vi "Station Detail Main.vi"(8 "error in (no error)":errorcluster, 11 "LineScan in":refnum<class "LineScan.lvclass">) -> (0 "error out":errorcluster, 2 "Station Out":T1=enum."ImformOut", 3 "LineScan out":refnum<class "LineScan.lvclass">)   [LabVIEW 2019, in "LineScan.lvclass"]
uses:
  LineScan.lvclass
  Ctrl/Station Action.ctl
  Ctrl/ProjectStepSelect.ctl
  Ctrl/StationCmdSelect.ctl
  Ctrl/Auto Inspection Station Name2.ctl
  Ctrl/Auto Inspection Data Name.ctl
  Ctrl/S2 Station IO.ctl
  Ctrl/MeasureDisplayTab.ctl
  Ctrl/Table Save.ctl
  Ctrl/ModbusCmd.ctl
  Ctrl/S2 Station Input.ctl
  Global/Process Global.vi
  LLB/Commonly VI/Main Glb.vi
  Ctrl/ProjectCmdStep.ctl
  BarcodeScan/Ctl/Board Scan IO.ctl
  Laser Detect/Ctl/S11 Station IO.ctl
  LLB/Commonly VI.lvlib
panel:
  out "data":dbl
  out "data 2":bool
  out "Array":string[](array[string])
  out "Blue Scan receive":string
  out "S1 ChkSum":string
  out "S1 ToolStringOut":string
  out "ToolStringOut_P1_2":string
  out "ToolStringOut_P1":string
  out "Initial_ChkSum":string
  out "ToolStringOut_Init":string
  out "CurrentCmd 2":string
  out "retry次數 2":string[](array[string])
  out "Retry 2":i32
  out "Program1 receive 2":string
  out "Initial receive 2":string
  out "T2 buffer":string
  out "T2 μA":dbl format="%#_6f"
  out "T1 μA":dbl format="%#_6f"
  out "T1 buffer":string
  out "S2 receive":string
  out "Blue Scan2 receive":string
  out "S1 receive":string
  out "Initial receive":string
  out "CurrentCmd":string
  out "Act Step":i32
  out "present":i32
  out "format receive":string
  out "Retry":i32
  out "subarray":string[](array[string])
  out "retry次數":string[](array[string])
  in  "Table Control":string[][](table)=[["PCBA BARCODE", ""], ["硬體(Tool初始化)", ""], ["company(Tool初始化)", ""], ["耗電流 uA(電流表)", "T"], ["電池負載電壓", "T"], ["晶片ID(Tool FORMAT)", "F"], ["雷雕ID(TOOl scan、藍芽接收器)", "S"], ["Format(Tool FORMAT)", "F"], ["Programe(Tool Programe)", "P"]]
  out "Numeric":dbl
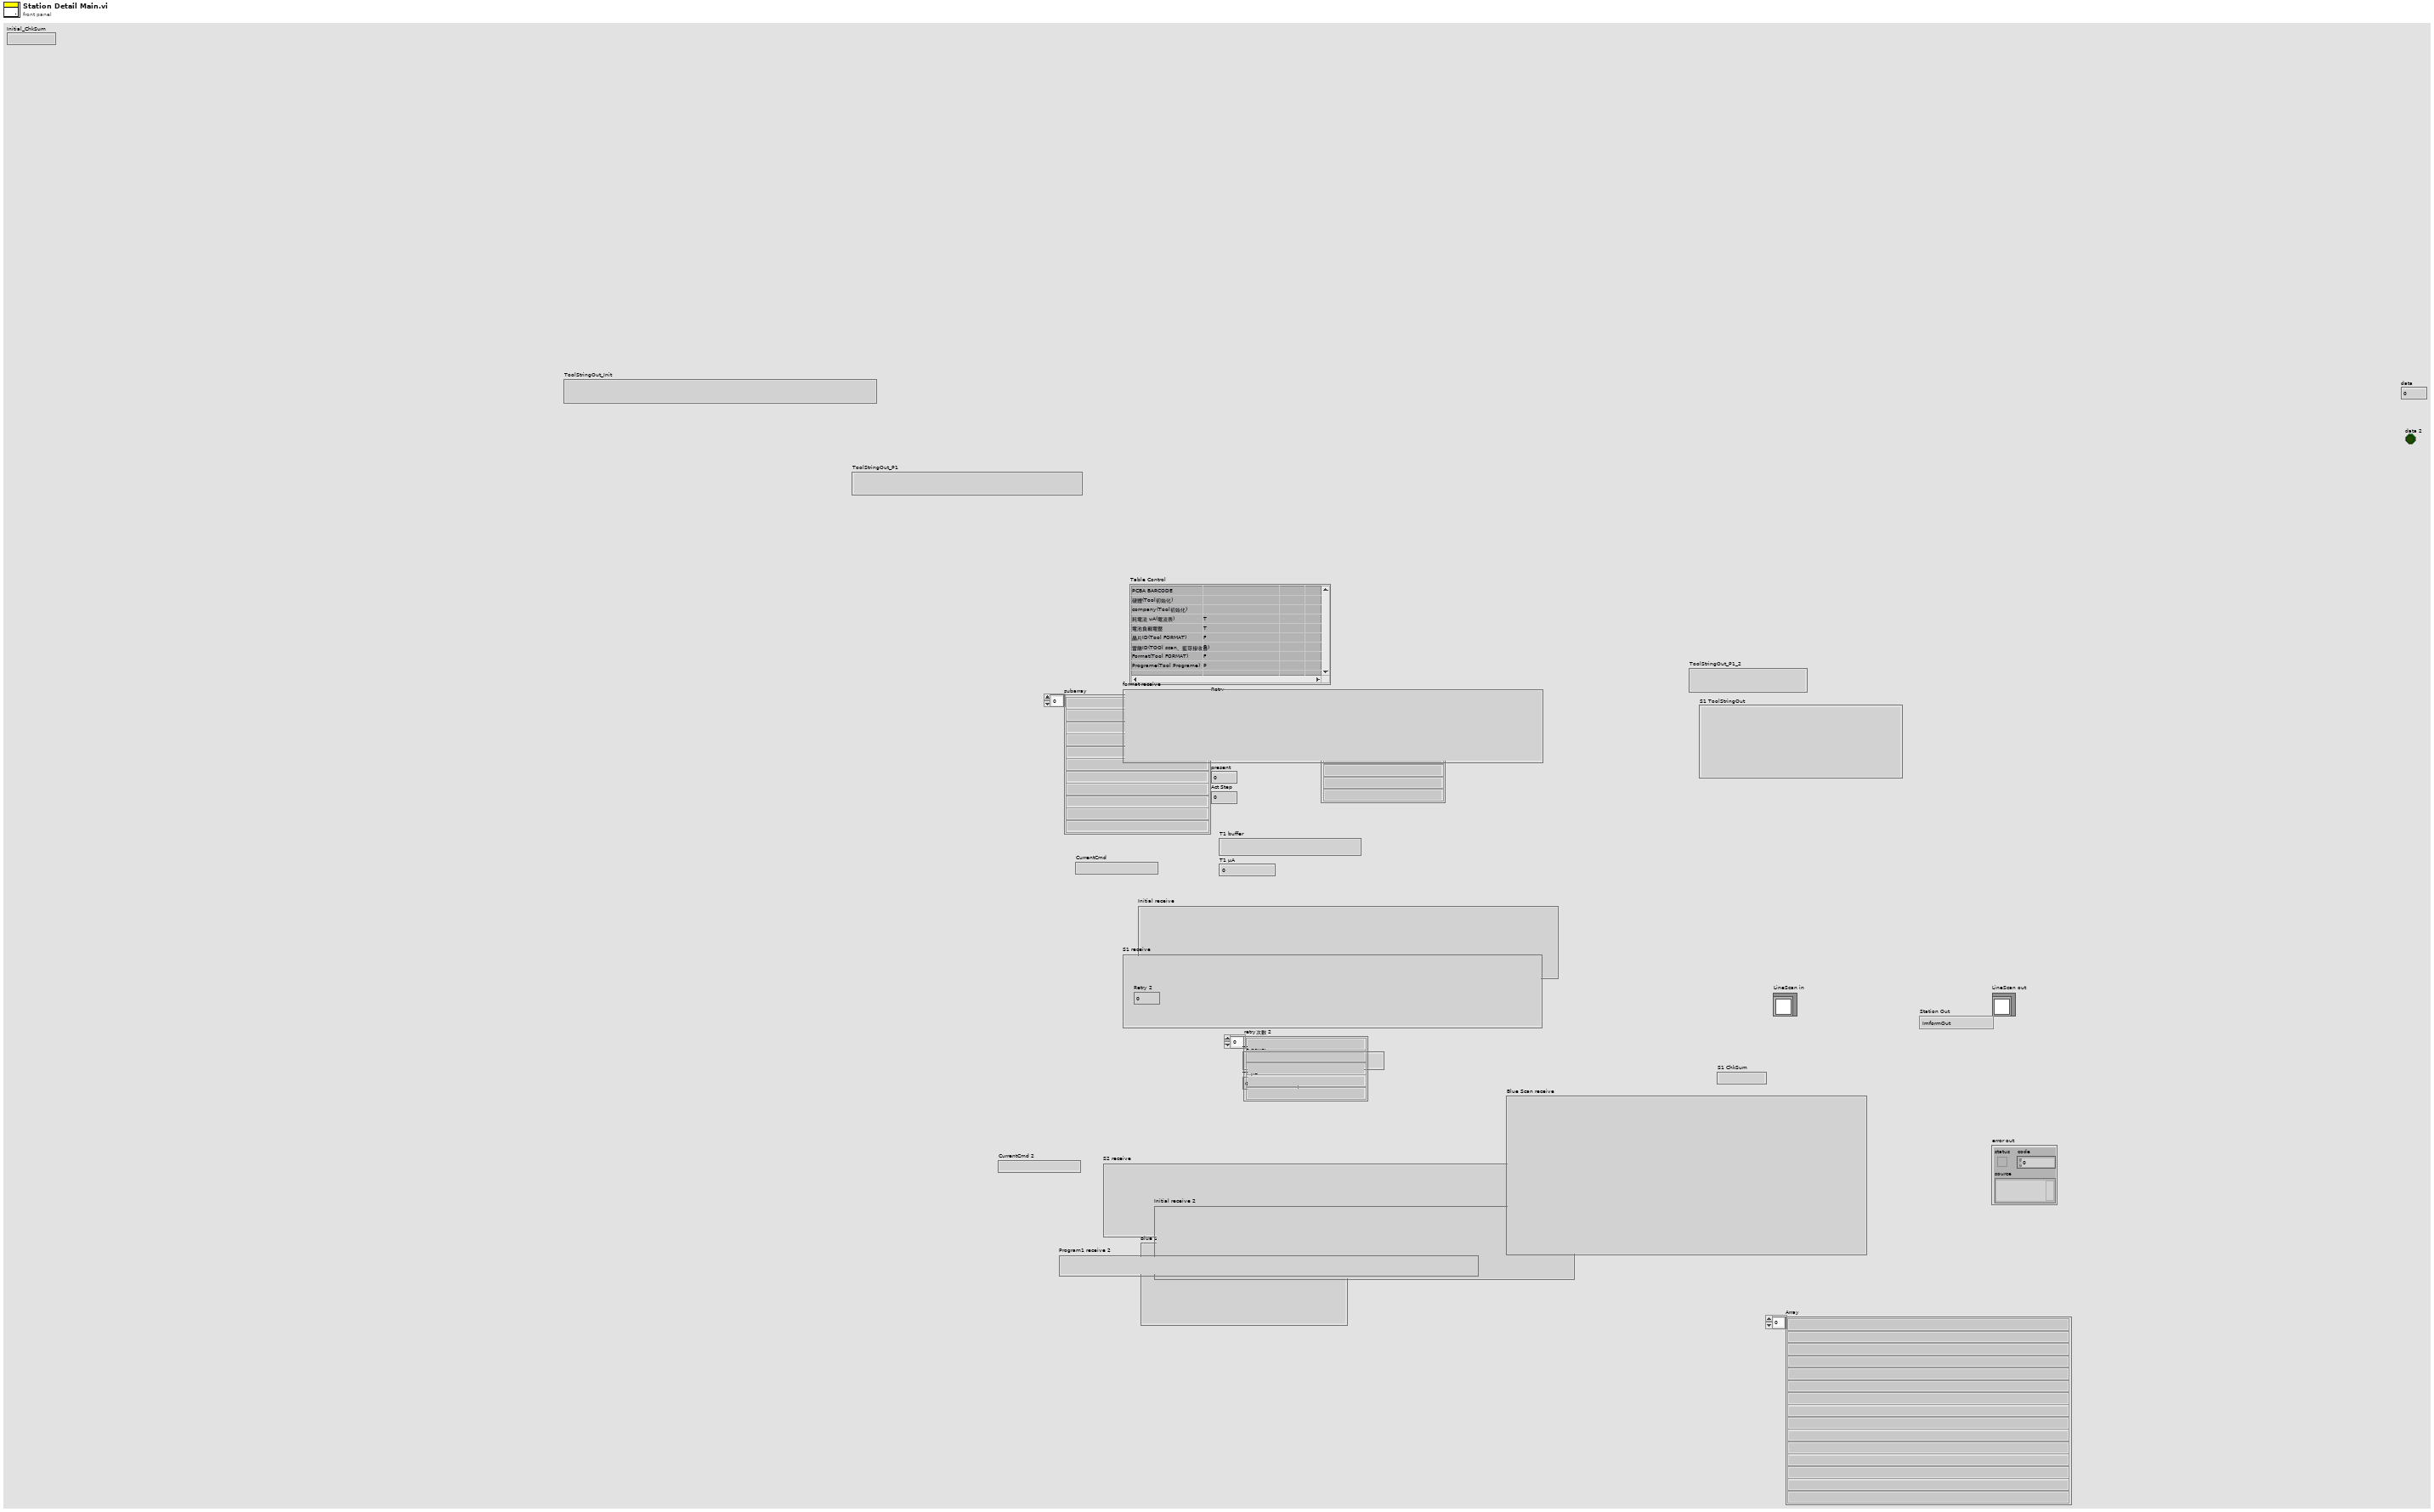
[diagram p1: front panel]
types:
  T1 = typedef "Station Action.ctl" = enum16{"Wait Item In", "Dectect Action", "ImformOut"}
  T2 = cluster{"starting address":u16, "number of inputs":u16, "Sat Coils":bool[], "Holding Registers":u16[]}
  T3 = typedef "ModbusCmd.ctl" = enum16{"Connect", "Disconnect", "Init", "Fetch Basic Objects", "Fetch Input Refisters", "Fetch Discrete Inputs", "Set Coils", "Set Holding Registers", "Write Single Holding", "Exit"}
  T4 = typedef "Board Scan IO.ctl" = enum16{"S1 Barcode Scan", "S1 載盤條碼比對OK", "S1 載盤條碼比對NG", "S1PLC 條碼可讀取訊號", "S1備用_04", "S1備用_05", "S1備用_06", "S1備用_07", "S1備用_08", "S1 發送條碼完成"}
  T5 = typedef "S2 Station IO.ctl" = enum16{"S2站PC動作中_20", "電流量測完成產品OK_21", "電流量測完成產品NG_22", "S2站Format 執行_23", "S2 Format OK_24", "S2 Format NG_25", "S2站燒入執行_26", "S2站燒入OK_27", "S2站燒入NG_28", "S2站動作完成_29", "S3 PC動作中_30", "S3 Format 此站執行_31", "S3 Format OK_32", "S3 Format NG_33", "S3 燒入程式 此站執行_34", "S3 燒入程式 OK_35", "S3 燒入程式 NG_36", "S3 備用_37", "S3 備用_38", "S3 動作完成_39", "S4 PC動作中_40", "S4 量測完成 產品正常_41", "S4 量測完成 產品NG_42", "S4 Format 此站執行_43", "S4 Format OK_44", "S4 Format NG_45", "S4 燒入 此站不執行_46", "S4 燒入程式 OK_47", "S4 燒入程式 NG_48", "S4 藍芽Scan OK_49", "S4 藍芽Scan NG_50", "S4 動作完成_51", "給PLC要量電流訊號", "給PLC要量電壓訊號"}
  T6 = typedef "S11 Station IO.ctl" = enum16{"S11雷射測量動作中", "S11雷射測點1完成", "S11雷射測點2完成", "S11雷測測量OK", "S11雷測測量NG", "S11雷測測量重測", "S11備用_6", "S11備用_7", "S11備用_8", "S11雷射測高完成"}
  T7 = typedef "StationCmdSelect.ctl" = enum16{"Action", "Command", "Return", "DTime", "Retry"}
  T8 = typedef "Auto Inspection Data Name.ctl" = enum16{"LocalRun", "ItemSN(TimeCode)", "CurrentAction", "Error", "Data", "OKNG", "電壓值", "電壓值判斷", "電流值", "電流值判斷", "Laser1 Data", "Laser2 Data", "Laser OKNG", "StationNO"}
  T9 = typedef "Auto Inspection Station Name2.ctl" = enum16{"S1Barcode", "S2Measure", "S3Measure", "S4Measure", "S5Measure", "S11_LaserCheck", "S8_Vision AI"}
  T10 = typedef "Table Save.ctl" = enum16{"initial", "Add", "Write", "Replace", "Delete", "REad", "RedTable", "Load"}
  T11 = typedef "MeasureDisplayTab.ctl" = enum16{"Tray Barcode", "PCBA BARCODE", "硬體(Tool初始化)", "company(Tool初始化)", "耗電流 uA(電流表)", "電池負載電壓", "晶片ID(Tool FORMAT)", "雷雕ID(TOOl scan、藍芽接收器)", "Format(Tool FORMAT)", "Programe(Tool Programe)", "MAC(藍芽接收器)", "ID(藍芽接收器)", "KPA(藍芽接收器)", "溫度(藍芽接收器)", "SENSOR電池電壓(藍芽接收器)", "RSSI(藍芽接收器)", "SensorType_315(FSK scan)", "FSKsnVol_315(FSK scan)", "FSKscanl_315(FSK scan)", "P_315(FSK scan)", "T_315(FSK scan)", "SensorType_433(ASK scan)", "ASKsnVol_433(ASK scan)", "ASKscan_433(ASK scan)", "P_433(ASK scan)", "T_433(ASK scan)", "測高Data"}
  T12 = typedef "S2 Station Input.ctl" = enum16{"00PLC Alive clock", "01PLC狀態(手動)", "02PLC狀態(自動)", "03PLC Alarm", "04備用", "05備用", "06備用", "07備用", "08備用", "09備用", "10載盤有料for條碼", "11_備用", "12_備用", "13_備用", "14_備用", "15_備用", "16_備用", "17_備用", "18_備用", "19_備用", "20_載盤有料訊號ForS2站", "21_PLC下達可測電流訊號", "22_PLC下達可測電壓訊號"}
  T13 = typedef "ProjectStepSelect.ctl" = enum16{"ProjectName", "Name", "Initial", "Reset", "Format", "Program1", "Program2", "Scan", "Finish", "MToolWork", "DataCheck", "DataSave", "OutputPLC", "WaitInputS1", "WaitInputOff"}
  T14 = typedef "ProjectCmdStep.ctl" = enum16{"Project Name", "commamd1", "commamd2", "commamd3", "wat time1", "return1", "return2", "return3", "wat time2", "over time", "retry"}
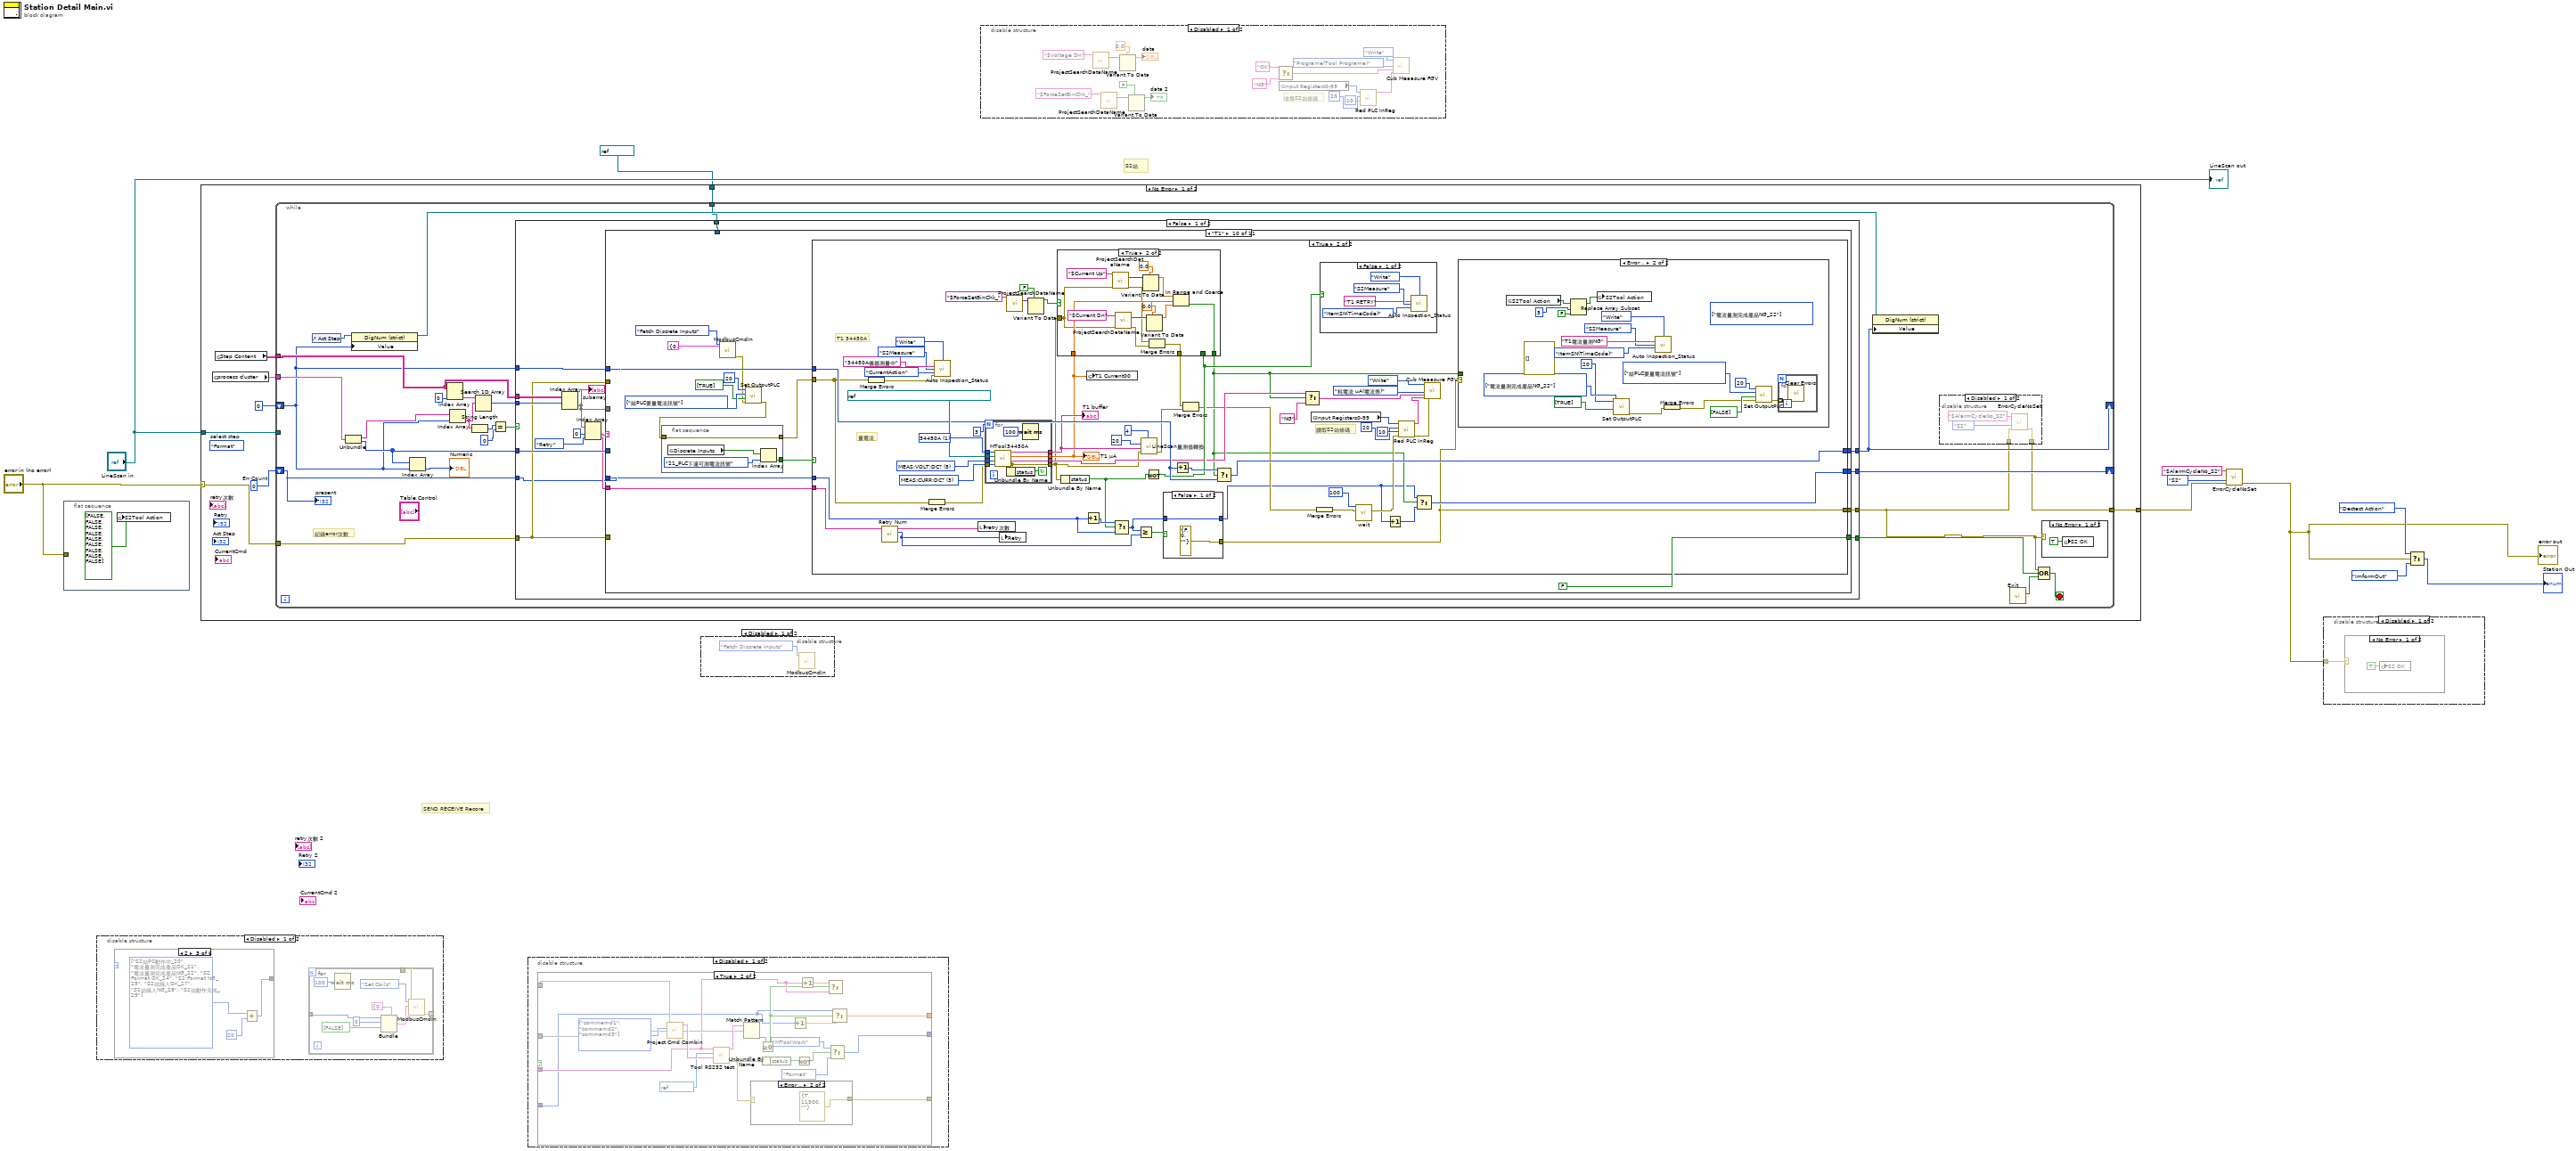
[diagram p0: block diagram]
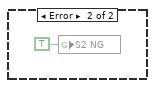
[diagram p2: hidden frame]
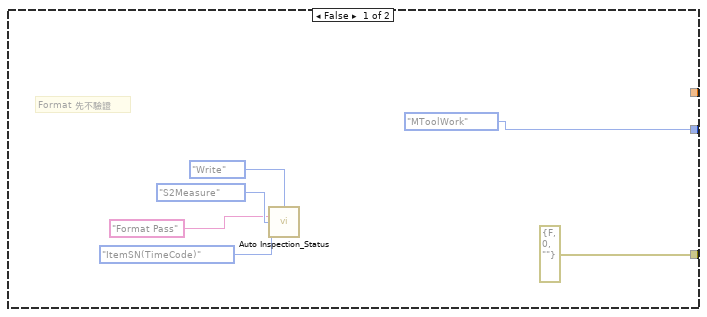
[diagram p6: hidden frame]
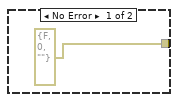
[diagram p7: hidden frame]
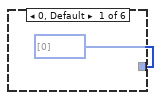
[diagram p9: hidden frame]
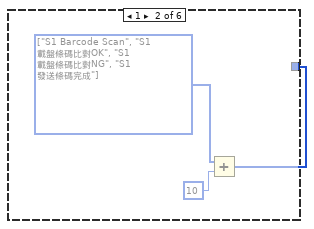
[diagram p10: hidden frame]
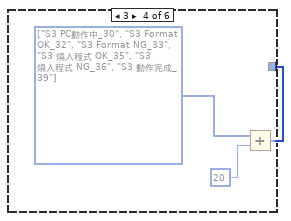
[diagram p11: hidden frame]
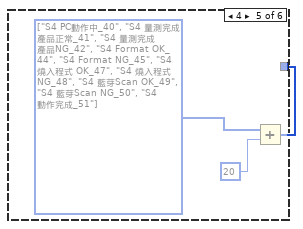
[diagram p12: hidden frame]
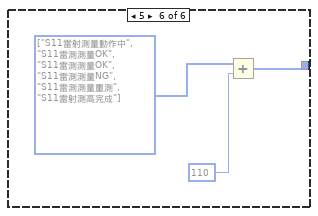
[diagram p13: hidden frame]
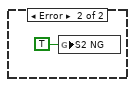
[diagram p15: hidden frame]
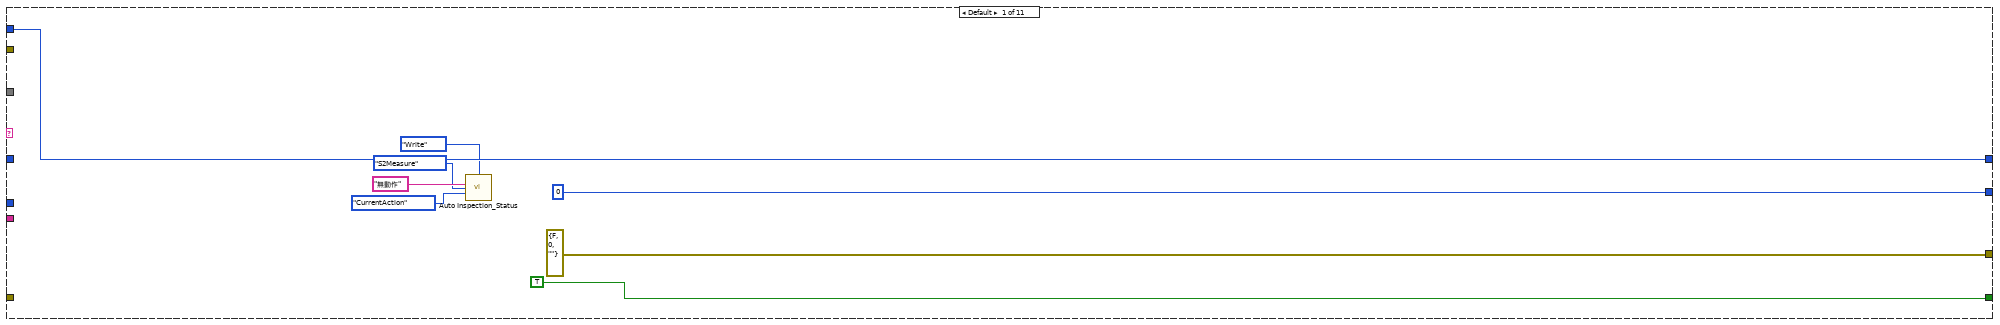
[diagram p17: hidden frame]
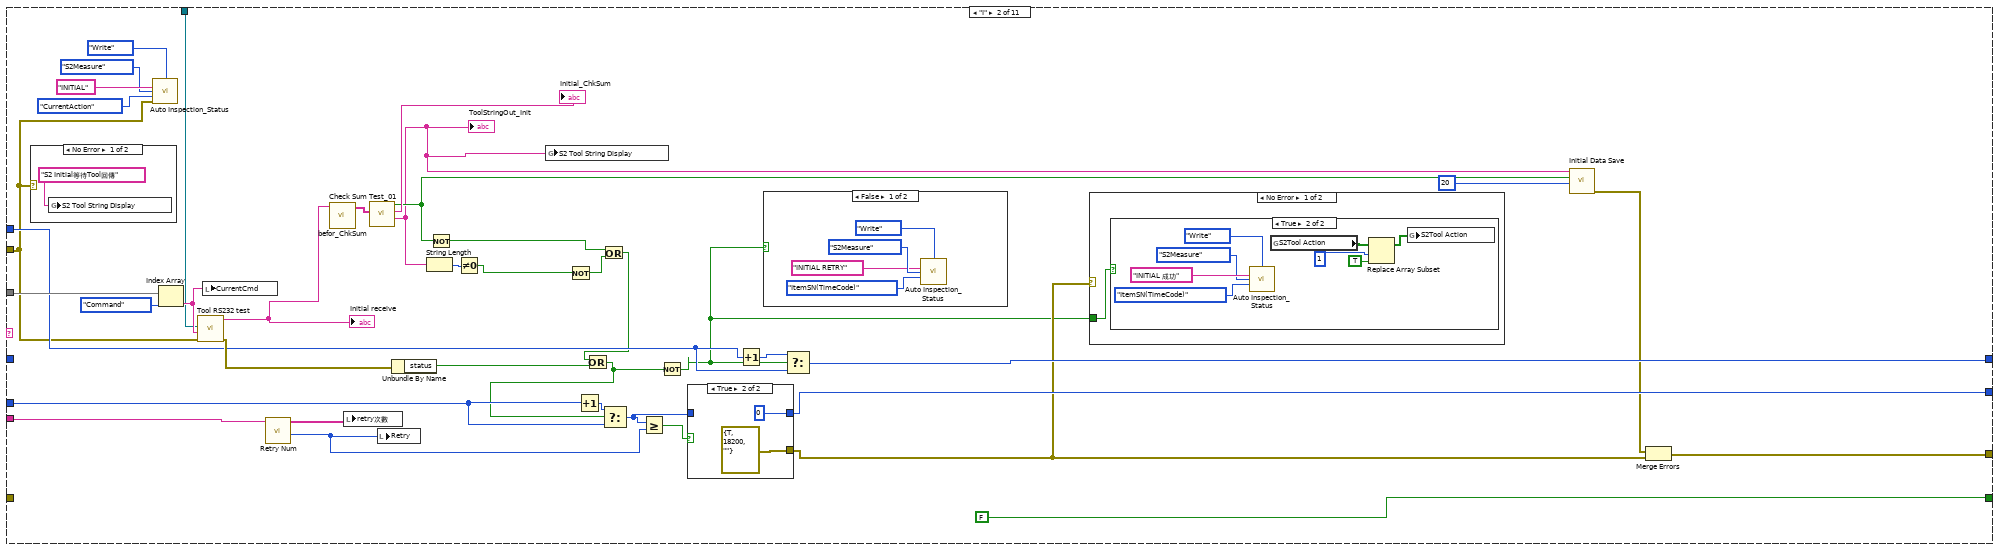
[diagram p18: hidden frame]
diagram:
  # "S2站"
  # "SEND RECEIVE Recore"
  n1 = flat-sequence {
    tunnel: "error in (no error)" -> [_]
    frame #0 {
      n2 = global write "Process Global.vi" "S2Tool Action"(bool[] [FALSE, FALSE, FALSE, FALSE, FALSE, FALSE, FALSE, FALSE, FALSE] ("S2Tool Action")) -> ()
    }
  }
  n3 = disable-structure shown="Disabled" {
    frame Disabled {
      n4 = case shown="2" {
        selector: _ -> [_ _ _ _ _ _]
        tunnel: [i32[] [0] w22 w25 w28 w31 w34] -> _
        frame 0, Default {
        }
        frame 1 {
          w24 = T4[] [enum."S1 Barcode Scan", enum."S1 載盤條碼比對OK", enum."S1 載盤條碼比對NG", enum."S1 發送條碼完成"] items=["S1 Barcode Scan", "S1 載盤條碼比對OK", "S1 載盤條碼比對NG", "S1PLC 條碼可讀取訊號", "S1備用_04", "S1備用_05", "S1備用_06", "S1備用_07", "S1備用_08", "S1 發送條碼完成"]
          n5 = Add(x=w24, y=10) -> (x+y=w22:i32[])
        }
        frame 2 {
          w26 = T5[] [enum."S2站PC動作中_20", enum."電流量測完成產品OK_21", enum."電流量測完成產品NG_22", enum."S2 Format OK_24", enum."S2 Format NG_25", enum."S2站燒入OK_27", enum."S2站燒入NG_28", enum."S2站動作完成_29"] items=["S2站PC動作中_20", "電流量測完成產品OK_21", "電流量測完成產品NG_22", "S2站Format 執行_23", "S2 Format OK_24", "S2 Format NG_25", "S2站燒入執行_26", "S2站燒入OK_27", "S2站燒入NG_28", "S2站動作完成_29", "S3 PC動作中_30", "S3 Format 此站執行_31", "S3 Format OK_32", "S3 Format NG_33", "S3 燒入程式 此站執行_34", "S3 燒入程式 OK_35", "S3 燒入程式 NG_36", "S3 備用_37", "S3 備用_38", "S3 動作完成_39", "S4 PC動作中_40", "S4 量測完成 產品正常_41", "S4 量測完成 產品NG_42", "S4 Format 此站執行_43", "S4 Format OK_44", "S4 Format NG_45", "S4 燒入 此站不執行_46", "S4 燒入程式 OK_47", "S4 燒入程式 NG_48", "S4 藍芽Scan OK_49", "S4 藍芽Scan NG_50", "S4 動作完成_51", "給PLC要量電流訊號", "給PLC要量電壓訊號"]
          n6 = Add(x=w26, y=20) -> (x+y=w25:i32[])
        }
        frame 3 {
          w29 = T5[] [enum."S3 PC動作中_30", enum."S3 Format OK_32", enum."S3 Format NG_33", enum."S3 燒入程式 OK_35", enum."S3 燒入程式 NG_36", enum."S3 動作完成_39"] items=["S2站PC動作中_20", "電流量測完成產品OK_21", "電流量測完成產品NG_22", "S2站Format 執行_23", "S2 Format OK_24", "S2 Format NG_25", "S2站燒入執行_26", "S2站燒入OK_27", "S2站燒入NG_28", "S2站動作完成_29", "S3 PC動作中_30", "S3 Format 此站執行_31", "S3 Format OK_32", "S3 Format NG_33", "S3 燒入程式 此站執行_34", "S3 燒入程式 OK_35", "S3 燒入程式 NG_36", "S3 備用_37", "S3 備用_38", "S3 動作完成_39", "S4 PC動作中_40", "S4 量測完成 產品正常_41", "S4 量測完成 產品NG_42", "S4 Format 此站執行_43", "S4 Format OK_44", "S4 Format NG_45", "S4 燒入 此站不執行_46", "S4 燒入程式 OK_47", "S4 燒入程式 NG_48", "S4 藍芽Scan OK_49", "S4 藍芽Scan NG_50", "S4 動作完成_51", "給PLC要量電流訊號", "給PLC要量電壓訊號"]
          n7 = Add(x=w29, y=20) -> (x+y=w28:i32[])
        }
        frame 4 {
          w32 = T5[] [enum."S4 PC動作中_40", enum."S4 量測完成 產品正常_41", enum."S4 量測完成 產品NG_42", enum."S4 Format OK_44", enum."S4 Format NG_45", enum."S4 燒入程式 OK_47", enum."S4 燒入程式 NG_48", enum."S4 藍芽Scan OK_49", enum."S4 藍芽Scan NG_50", enum."S4 動作完成_51"] items=["S2站PC動作中_20", "電流量測完成產品OK_21", "電流量測完成產品NG_22", "S2站Format 執行_23", "S2 Format OK_24", "S2 Format NG_25", "S2站燒入執行_26", "S2站燒入OK_27", "S2站燒入NG_28", "S2站動作完成_29", "S3 PC動作中_30", "S3 Format 此站執行_31", "S3 Format OK_32", "S3 Format NG_33", "S3 燒入程式 此站執行_34", "S3 燒入程式 OK_35", "S3 燒入程式 NG_36", "S3 備用_37", "S3 備用_38", "S3 動作完成_39", "S4 PC動作中_40", "S4 量測完成 產品正常_41", "S4 量測完成 產品NG_42", "S4 Format 此站執行_43", "S4 Format OK_44", "S4 Format NG_45", "S4 燒入 此站不執行_46", "S4 燒入程式 OK_47", "S4 燒入程式 NG_48", "S4 藍芽Scan OK_49", "S4 藍芽Scan NG_50", "S4 動作完成_51", "給PLC要量電流訊號", "給PLC要量電壓訊號"]
          n8 = Add(x=w32, y=20) -> (x+y=w31:i32[])
        }
        frame 5 {
          w35 = T6[] [enum."S11雷射測量動作中", enum."S11雷測測量OK", enum."S11雷測測量OK", enum."S11雷測測量NG", enum."S11雷測測量重測", enum."S11雷射測高完成"] items=["S11雷射測量動作中", "S11雷射測點1完成", "S11雷射測點2完成", "S11雷測測量OK", "S11雷測測量NG", "S11雷測測量重測", "S11備用_6", "S11備用_7", "S11備用_8", "S11雷射測高完成"]
          n9 = Add(x=w35, y=110) -> (x+y=w34:i32[])
        }
      }
      n10 = for {
        tunnel: [w14] -> _ mode=indexing
        tunnel: _ -> [w13]
        tunnel: _ -> [w12] mode=indexing
        n11 = Wait (ms)(milliseconds to wait=100) -> ()  [unwired: 1 out]
        n12 = Bundle(cluster=T2 {"starting address"=0, "number of inputs"=0, "Sat Coils"=[], "Holding Registers"=[]} ("data"), "starting address"=w12, "number of inputs"=u16 0, "Sat Coils"=bool[] [FALSE]) -> (w17:T2)  [unwired: 1 in]
        n13 = call "ModbusCmdIn.vi"("error in (no error)"=w13, "data"=w17, "Enum"=ModbusCmd."Set Coils") -> ("error out"=w14:errorcluster)  [unwired: 8 in]
      }
    }
    frame Enabled {
    }
  }
  n14 = case shown="No Error" "error in (no error)" {
    selector: "error in (no error)" -> [w38 w854]
    tunnel: [w44 w854] -> w2
    tunnel: "LineScan in" -> [w43 _]
    tunnel: refnum<visa-resource-name> "COM1" ("VISA resource name") -> [w37 _]
    frame No Error {
      w39 = 0  # Err Count
      (unwired) ProjectStepSelect."Format"  # select step
      n15 = global read "Process Global.vi" "process cluster"() -> (w41:cluster{string[], i32[]})
      n16 = global read "Process Global.vi" "Step Content"() -> (w42:string[][])
      n17 = while {
        tunnel: [w45] -> w44
        shift-right: [w52] -> _
        shift-left: 0 -> [w53]
        tunnel: w43 -> [_]
        shift-right: [w49] -> _
        shift-left: w39 -> [w55]
        tunnel: w42 -> [w66]
        tunnel: w41 -> [w65]
        tunnel: w38 -> [w50]
        tunnel: w37 -> [w48]
        stop <- w67 stop-if-true
        # "紀錄error次數"
        n18 = control-ref of="Act Step"() -> (w54:refnum<vi>)
        n19 = Unbundle(w65) -> (w68:string[], w69:i32[])
        n20 = property class="DigNum (strict)"(reference=w54, "Value"=w53) -> (reference out=w51:refnum<vi>)  [unwired: 1 in, 1 out]
        n21 = Index Array(array=w69, index=w53) -> (element=→"Numeric":i32)
        n22 = Index Array(array=w66, index (col)=0 ("disabled index (col)")) -> (element=w63:string[])  [unwired: 1 in]
        n23 = Index Array(array=w68, index=w53) -> (element=w59:string)
        n24 = String Length(string=w59) -> (length=w60:i32)
        n25 = Search 1D Array(1D array=w63, element=w59) -> (index of element=w62:i32)  [unwired: 1 in]
        n26 = Equal?(x=w60, y=0) -> (x = y?=w57:bool)
        n27 = case shown="False" w57 {
          tunnel: w69 -> [w92 _]
          tunnel: w66 -> [w91 _]
          tunnel: w62 -> [w90 _]
          tunnel: [w81 TRUE] -> w56
          tunnel: [w83 errorcluster {"status"=FALSE, "code"=0, "source"=""} ("error constant")] -> w46
          tunnel: w53 -> [w85 _]
          tunnel: [w84 w851] -> w52
          tunnel: w55 -> [w79 _]
          tunnel: w50 -> [w80 _]
          tunnel: [w78 w851] -> w49
          tunnel: w48 -> [w77 _]
          frame False {
            n28 = Index Array(array=w91, index (row)=w90) -> (element=w86:string[])  [unwired: 1 in]
            "subarray" <- w86
            n29 = Index Array(array=w86, index #1=0 ("index"), index #2=StationCmdSelect."Retry") -> (element #1=w88:string, element #2=w87:string)
            n30 = case shown="\"T1\"" w88 {
              tunnel: w92 -> [_ _ _ _ _ _ _ _ w583 _ _]
              tunnel: w87 -> [_ w129 w176 w244 w340 w394 w493 w537 _ w599 w753]
              tunnel: w86 -> [_ w130 w177 w243 w342 w397 w492 w538 _ _ _]
              tunnel: w85 -> [w100 w113 w178 w239 w341 w396 w468 w540 w578 w598 w755]
              tunnel: [w100 w128 w175 w241 w339 w393 w494 w536 w577 w597 w754] -> w84
              tunnel: [errorcluster {"status"=FALSE, "code"=0, "source"=""} ("error constant") w106 w168 w227 w300 w390 w485 w533 errorcluster {"status"=FALSE, "code"=0, "source"=""} ("error constant") w596 w752] -> w83
              tunnel: [TRUE FALSE FALSE FALSE FALSE FALSE FALSE FALSE FALSE FALSE FALSE] -> w81
              tunnel: w80 -> [_ _ _ _ _ _ _ _ _ _ _]
              tunnel: w80 -> [_ w102 w167 w218 w298 w389 w456 w539 _ _ _]
              tunnel: w79 -> [_ w121 w171 w221 w324 w395 w470 w517 _ w594 w751]
              tunnel: [0 ("Err Count") w122 w172 w222 w325 w392 w471 w518 0 ("Err Count") w595 w750] -> w78
              tunnel: w77 -> [_ w120 w169 w220 w314 w398 w469 w516 _ _ _]
              frame Default {
                n31 = call "Auto Inspection_Status.vi"("Action"=enum16{"Initial", "Write", "Read"}."Write", "DataIn"="無動作", "Station"=Auto_Inspection_Station_Name2."S2Measure", "Data"=Auto_Inspection_Data_Name."CurrentAction") -> ()  [unwired: 9 in, 3 out]
              }
              frame "I" {
                n32 = case shown="No Error" w102 {
                  frame No Error {
                    n33 = global write "Process Global.vi" "S2 Tool String Display"("S2 Initial等待Tool回傳" ("S2 Tool String Display")) -> ()
                  }
                  frame Error {
                  }
                }
                n34 = call "Auto Inspection_Status.vi"("Action"=enum16{"Initial", "Write", "Read"}."Write", "DataIn"="INITIAL", "Station"=Auto_Inspection_Station_Name2."S2Measure", "Data"=Auto_Inspection_Data_Name."CurrentAction", "error in"=w102) -> ()  [unwired: 8 in, 3 out]
                n35 = Index Array(array=w130, index=StationCmdSelect."Command") -> (element=w132:string)
                n36 = call "Tool RS232 test.vi"("error in (no error)"=w102, "Cmd In"=w132, "VISA resource name"=w120) -> ("error out"=w139:errorcluster, "receive string"=w105:string)  [unwired: 7 in]
                "Initial receive" <- w105
                n37 = local write "CurrentCmd"(w132) -> ()
                n38 = call "Retry Num.vi"("String"=w129) -> ("Numeric"=w136:i32, "retry次數"=w133:string[])  [unwired: 9 in]
                n39 = call "befor_ChkSum.vi"("ToolString Input"=w105) -> ("Array"=w115:string[])  [unwired: 9 in, 1 out]
                n40 = local write "retry次數"(w133) -> ()
                n41 = call "Check Sum Test_01.vi"("Array"=w115) -> ("ToolStringOut_01"=w104:string, "ChkSum"=→"Initial_ChkSum":string, "x = y?"=w109:bool)  [unwired: 8 in]
                "ToolStringOut_Init" <- w104
                n42 = local write "Retry"(w136) -> ()
                n43 = Unbundle By Name(w139) -> ("status"=w112:bool)
                n44 = String Length(string=w104) -> (length=w118:i32)
                n45 = Not(x=w109) -> (.not. x?=w116:bool)
                n46 = Not Equal To 0?(x=w118) -> (x != 0?=w119:bool)
                n47 = global write "Process Global.vi" "S2 Tool String Display"(w104) -> ()
                n48 = Not(x=w119) -> (.not. x?=w117:bool)
                n49 = Increment(x=w121) -> (x+1=w137:i32)
                n50 = Or(x=w116, y=w117) -> (x .or. y?=w111:bool)
                n51 = Or(x=w111, y=w112) -> (x .or. y?=w110:bool)
                n52 = Select(t=w137, s=w110, f=w121) -> (s? t:f=w134:i32)
                n53 = Greater Or Equal?(x=w134, y=w136) -> (x >= y?=w135:bool)
                n54 = Not(x=w110) -> (.not. x?=w101:bool)
                n55 = case shown="True" w135 {
                  tunnel: [errorcluster {"status"=FALSE, "code"=0, "source"=""} ("error constant") errorcluster {"status"=TRUE, "code"=18200, "source"=""} ("error constant")] -> w103
                  tunnel: w134 -> [w162 _]
                  tunnel: [w162 0] -> w122
                  frame False {
                  }
                  frame True {
                  }
                }
                n56 = Increment(x=w113) -> (x+1=w138:i32)
                n57 = case shown="False" w101 {
                  frame False {
                    n58 = call "Auto Inspection_Status.vi"("Action"=enum16{"Initial", "Write", "Read"}."Write", "DataIn"="INITIAL RETRY", "Station"=Auto_Inspection_Station_Name2."S2Measure", "Data"=Auto_Inspection_Data_Name."ItemSN(TimeCode)") -> ()  [unwired: 9 in, 3 out]
                  }
                  frame True {
                  }
                }
                n59 = Select(t=w138, s=w101, f=w113) -> (s? t:f=w128:i32)
                n60 = case shown="No Error" w103 {
                  tunnel: w101 -> [w145 _]
                  frame No Error {
                    n61 = case shown="True" w145 {
                      frame False {
                      }
                      frame True {
                        n62 = call "Auto Inspection_Status.vi"("Action"=enum16{"Initial", "Write", "Read"}."Write", "DataIn"="INITIAL 成功", "Station"=Auto_Inspection_Station_Name2."S2Measure", "Data"=Auto_Inspection_Data_Name."ItemSN(TimeCode)") -> ()  [unwired: 9 in, 3 out]
                        n63 = global read "Process Global.vi" "S2Tool Action"() -> (w149:bool[])
                        n64 = Replace Array Subset(array=w149, new element=TRUE ("new element/subarray"), index=1) -> (w146:bool[])
                        n65 = global write "Process Global.vi" "S2Tool Action"(w146) -> ()
                      }
                    }
                  }
                  frame Error {
                    n66 = call "Auto Inspection_Status.vi"("Action"=enum16{"Initial", "Write", "Read"}."Write", "DataIn"="INITIAL 失敗 ", "Station"=Auto_Inspection_Station_Name2."S2Measure", "Data"=Auto_Inspection_Data_Name."ItemSN(TimeCode)") -> ()  [unwired: 9 in, 3 out]
                    n67 = global read "Process Global.vi" "S2Tool Action"() -> (w157:bool[])
                    n68 = Replace Array Subset(array=w157, new element=FALSE ("new element/subarray"), index=1) -> (w154:bool[])
                    n69 = global write "Process Global.vi" "S2Tool Action"(w154) -> ()
                  }
                }
                n70 = call "Initial Data Save.vi"("index"=20, "OK and NG"=w109, "String In"=w104) -> ("error out"=w107:errorcluster)  [unwired: 8 in]
                n71 = Merge Errors(w107, w103) -> (w106:errorcluster)
              }
              frame "R" {
                n72 = call "Auto Inspection_Status.vi"("Action"=enum16{"Initial", "Write", "Read"}."Write", "DataIn"="RESET", "Station"=Auto_Inspection_Station_Name2."S2Measure", "Data"=Auto_Inspection_Data_Name."CurrentAction", "error in"=w167) -> ()  [unwired: 8 in, 3 out]
                n73 = call "Retry Num.vi"("String"=w176) -> ("Numeric"=w186:i32, "retry次數"=w185:string[])  [unwired: 9 in]
                n74 = Index Array(array=w177, index=StationCmdSelect."Command") -> (element=w184:string)
                n75 = local write "retry次數"(w185) -> ()
                n76 = call "Tool RS232 test.vi"("error in (no error)"=w167, "Cmd In"=w184, "VISA resource name"=w169) -> ("error out"=w190:errorcluster, "receive string"=→"Initial receive 2":string)  [unwired: 7 in]
                n77 = local write "CurrentCmd"(w184) -> ()
                n78 = local write "Retry"(w186) -> ()
                n79 = Unbundle By Name(w190) -> ("status"=w188:bool)
                n80 = Increment(x=w171) -> (x+1=w187:i32)
                n81 = Not(x=w188) -> (.not. x?=w166:bool)
                n82 = Select(t=w187, s=w188, f=w171) -> (s? t:f=w173:i32)
                n83 = Greater Or Equal?(x=w173, y=w186) -> (x >= y?=w170:bool)
                n84 = case shown="True" w170 {
                  tunnel: [errorcluster {"status"=FALSE, "code"=0, "source"=""} ("error constant") errorcluster {"status"=TRUE, "code"=18207, "source"=""} ("error constant")] -> w168
                  tunnel: w173 -> [w213 w215]
                  tunnel: [w213 w215] -> w172
                  frame False {
                  }
                  frame True {
                  }
                }
                n85 = case shown="False" w166 {
                  frame False {
                    n86 = call "Auto Inspection_Status.vi"("Action"=enum16{"Initial", "Write", "Read"}."Write", "DataIn"="RESET RETRY ", "Station"=Auto_Inspection_Station_Name2."S2Measure", "Data"=Auto_Inspection_Data_Name."ItemSN(TimeCode)") -> ()  [unwired: 9 in, 3 out]
                  }
                  frame True {
                  }
                }
                n87 = Increment(x=w178) -> (x+1=w189:i32)
                n88 = Select(t=w189, s=w166, f=w178) -> (s? t:f=w175:i32)
                n89 = case shown="No Error" w168 {
                  tunnel: w166 -> [w196 _]
                  frame No Error {
                    n90 = case shown="True" w196 {
                      frame False {
                      }
                      frame True {
                        n91 = call "Auto Inspection_Status.vi"("Action"=enum16{"Initial", "Write", "Read"}."Write", "DataIn"="RESET 成功 ", "Station"=Auto_Inspection_Station_Name2."S2Measure", "Data"=Auto_Inspection_Data_Name."ItemSN(TimeCode)") -> ()  [unwired: 9 in, 3 out]
                        n92 = global read "Process Global.vi" "S2Tool Action"() -> (w200:bool[])
                        n93 = Replace Array Subset(array=w200, new element=TRUE ("new element/subarray"), index=0) -> (w197:bool[])
                        n94 = global write "Process Global.vi" "S2Tool Action"(w197) -> ()
                      }
                    }
                  }
                  frame Error {
                    n95 = call "Auto Inspection_Status.vi"("Action"=enum16{"Initial", "Write", "Read"}."Write", "DataIn"="RESET 失敗 ", "Station"=Auto_Inspection_Station_Name2."S2Measure", "Data"=Auto_Inspection_Data_Name."ItemSN(TimeCode)") -> ()  [unwired: 9 in, 3 out]
                    n96 = global read "Process Global.vi" "S2Tool Action"() -> (w208:bool[])
                    n97 = Replace Array Subset(array=w208, new element=FALSE ("new element/subarray"), index=0) -> (w205:bool[])
                    n98 = global write "Process Global.vi" "S2Tool Action"(w205) -> ()
                  }
                }
              }
              frame "F" {
                # "SEND RECEIVE Recore"
                n99 = call "Retry Num.vi"("String"=w244) -> ("Numeric"=w235:i32, "retry次數"=w231:string[])  [unwired: 9 in]
                n100 = local write "retry次數"(w231) -> ()
                n101 = Index Array(array=w243, index=StationCmdSelect."Command") -> (element=w230:string)
                n102 = local write "Retry"(w235) -> ()
                n103 = call "Tool RS232 test.vi"("error in (no error)"=w218, "Cmd In"=w230, "VISA resource name"=w220) -> ("error out"=w240:errorcluster, "receive string"=→"format receive":string)  [unwired: 7 in]
                n104 = local write "CurrentCmd"(w230) -> ()
                n105 = Unbundle By Name(w240) -> ("status"=w237:bool)
                n106 = Not(x=w237) -> (.not. x?=w217:bool)
                n107 = call "Auto Inspection_Status.vi"("Action"=enum16{"Initial", "Write", "Read"}."Write", "DataIn"="FORMAT", "Station"=Auto_Inspection_Station_Name2."S2Measure", "Data"=Auto_Inspection_Data_Name."CurrentAction", "error in"=w218) -> ()  [unwired: 8 in, 3 out]
                n108 = Increment(x=w221) -> (x+1=w236:i32)
                n109 = Select(t=w236, s=w237, f=w221) -> (s? t:f=w232:i32)
                n110 = Increment(x=w239) -> (x+1=w238:i32)
                n111 = Greater Or Equal?(x=w232, y=w235) -> (x >= y?=w234:bool)
                n112 = Select(t=w238, s=w217, f=w239) -> (s? t:f=w241:i32)
                n113 = case shown="True" w234 {
                  tunnel: [errorcluster {"status"=FALSE, "code"=0, "source"=""} ("error constant") errorcluster {"status"=TRUE, "code"=18201, "source"=""} ("error constant")] -> w219
                  tunnel: w232 -> [w289 _]
                  tunnel: [w289 0] -> w222
                  frame False {
                  }
                  frame True {
                  }
                }
                n114 = case shown="False" w217 {
                  frame False {
                    n115 = call "Auto Inspection_Status.vi"("Action"=enum16{"Initial", "Write", "Read"}."Write", "DataIn"="FORMAT RETRY ", "Station"=Auto_Inspection_Station_Name2."S2Measure", "Data"=Auto_Inspection_Data_Name."ItemSN(TimeCode)") -> ()  [unwired: 9 in, 3 out]
                  }
                  frame True {
                  }
                }
                n116 = case shown="No Error" w219 {
                  tunnel: [w250 w286] -> w228
                  tunnel: w217 -> [w249 _]
                  frame No Error {
                    n117 = case shown="True" w249 {
                      tunnel: [_ w267] -> w250
                      frame False {
                      }
                      frame True {
                        w268 = T5[] [enum."S2站Format 執行_23", enum."S2 Format OK_24"] items=["S2站PC動作中_20", "電流量測完成產品OK_21", "電流量測完成產品NG_22", "S2站Format 執行_23", "S2 Format OK_24", "S2 Format NG_25", "S2站燒入執行_26", "S2站燒入OK_27", "S2站燒入NG_28", "S2站動作完成_29", "S3 PC動作中_30", "S3 Format 此站執行_31", "S3 Format OK_32", "S3 Format NG_33", "S3 燒入程式 此站執行_34", "S3 燒入程式 OK_35", "S3 燒入程式 NG_36", "S3 備用_37", "S3 備用_38", "S3 動作完成_39", "S4 PC動作中_40", "S4 量測完成 產品正常_41", "S4 量測完成 產品NG_42", "S4 Format 此站執行_43", "S4 Format OK_44", "S4 Format NG_45", "S4 燒入 此站不執行_46", "S4 燒入程式 OK_47", "S4 燒入程式 NG_48", "S4 藍芽Scan OK_49", "S4 藍芽Scan NG_50", "S4 動作完成_51", "給PLC要量電流訊號", "給PLC要量電壓訊號"]
                        # "收尋S2站條碼"
                        n118 = global read "Main Glb.vi" "Input Registers0-99"() -> (w255:u16[])
                        n119 = call "Set OutputPLC.vi"("Address In"=20, "Array 2"=w268, "Sat Coils"=bool[] [TRUE]) -> ("Error Out"=w267:errorcluster[])  [unwired: 7 in]
                        n120 = global read "Process Global.vi" "S2Tool Action"() -> (w262:bool[])
                        n121 = call "Red PLC InReg.vi"("length"=10, "index"=20, "Input Registers Arr"=w255) -> ("Rad In Reg"=w258:string)  [unwired: 7 in, 1 out]
                        n122 = call "Cub Meaasure FGV.vi"("Action"=Table_Save."Write" ("Enum"), "Save Index"=MeasureDisplayTab."Format(Tool FORMAT)", "DataIn"="OK", "SN"=w258) -> ()  [unwired: 8 in, 8 out]
                        n123 = Replace Array Subset(array=w262, new element=TRUE ("new element/subarray"), index=2) -> (w259:bool[])
                        n124 = global write "Process Global.vi" "S2Tool Action"(w259) -> ()
                        n125 = call "Auto Inspection_Status.vi"("Action"=enum16{"Initial", "Write", "Read"}."Write", "DataIn"="FORMAT完成", "Station"=Auto_Inspection_Station_Name2."S2Measure", "Data"=Auto_Inspection_Data_Name."ItemSN(TimeCode)") -> ()  [unwired: 9 in, 3 out]
                      }
                    }
                  }
                  frame Error {
                    w288 = T5[] [enum."S2站Format 執行_23", enum."S2 Format NG_25"] items=["S2站PC動作中_20", "電流量測完成產品OK_21", "電流量測完成產品NG_22", "S2站Format 執行_23", "S2 Format OK_24", "S2 Format NG_25", "S2站燒入執行_26", "S2站燒入OK_27", "S2站燒入NG_28", "S2站動作完成_29", "S3 PC動作中_30", "S3 Format 此站執行_31", "S3 Format OK_32", "S3 Format NG_33", "S3 燒入程式 此站執行_34", "S3 燒入程式 OK_35", "S3 燒入程式 NG_36", "S3 備用_37", "S3 備用_38", "S3 動作完成_39", "S4 PC動作中_40", "S4 量測完成 產品正常_41", "S4 量測完成 產品NG_42", "S4 Format 此站執行_43", "S4 Format OK_44", "S4 Format NG_45", "S4 燒入 此站不執行_46", "S4 燒入程式 OK_47", "S4 燒入程式 NG_48", "S4 藍芽Scan OK_49", "S4 藍芽Scan NG_50", "S4 動作完成_51", "給PLC要量電流訊號", "給PLC要量電壓訊號"]
                    # "收尋S2站條碼"
                    n126 = global read "Main Glb.vi" "Input Registers0-99"() -> (w274:u16[])
                    n127 = call "Set OutputPLC.vi"("Address In"=20, "Array 2"=w288, "Sat Coils"=bool[] [TRUE]) -> ("Error Out"=w286:errorcluster[])  [unwired: 7 in]
                    n128 = call "Red PLC InReg.vi"("length"=10, "index"=20, "Input Registers Arr"=w274) -> ("Rad In Reg"=w277:string)  [unwired: 7 in, 1 out]
                    n129 = global read "Process Global.vi" "S2Tool Action"() -> (w281:bool[])
                    n130 = call "Cub Meaasure FGV.vi"("Action"=Table_Save."Write" ("Enum"), "Save Index"=MeasureDisplayTab."Format(Tool FORMAT)", "DataIn"="NG", "SN"=w277) -> ()  [unwired: 8 in, 8 out]
                    n131 = call "Auto Inspection_Status.vi"("Action"=enum16{"Initial", "Write", "Read"}."Write", "DataIn"="FORMAT 失敗 ", "Station"=Auto_Inspection_Station_Name2."S2Measure", "Data"=Auto_Inspection_Data_Name."ItemSN(TimeCode)") -> ()  [unwired: 9 in, 3 out]
                    n132 = Replace Array Subset(array=w281, new element=FALSE ("new element/subarray"), index=2) -> (w278:bool[])
                    n133 = global write "Process Global.vi" "S2Tool Action"(w278) -> ()
                  }
                }
                n134 = Merge Errors(w228, w219) -> (w227:errorcluster)
              }
              frame "P1" {
                # "經過燒錄後第二次Tool回傳"
                # "下Cmd後第一次Tool回傳"
                # "收尋S2站條碼"
                n135 = case shown="No Error" w298 {
                  frame No Error {
                    n136 = global write "Process Global.vi" "S2 Tool String Display"("S2燒錄 等待Tool回傳" ("S2 Tool String Display")) -> ()
                  }
                  frame Error {
                  }
                }
                n137 = call "Retry Num.vi"("String"=w340) -> ("Numeric"=w348:i32, "retry次數"=w345:string[])  [unwired: 9 in]
                n138 = Index Array(array=w342, index=StationCmdSelect."Command") -> (element=w344:string)
                n139 = local write "retry次數"(w345) -> ()
                n140 = call "Tool RS232 test.vi"("error in (no error)"=w298, "Cmd In"=w344, "VISA resource name"=w314) -> ("error out"=w315:errorcluster, "receive string"=w316:string)  [unwired: 7 in]
                n141 = local write "CurrentCmd"(w344) -> ()
                n142 = local write "Retry"(w348) -> ()
                n143 = call "befor_ChkSum.vi"("ToolString Input"=w316) -> ("Array"=w317:string[])  [unwired: 9 in, 1 out]
                n144 = call "Check Sum Test_01.vi"("Array"=w317) -> ("ToolStringOut_01"=w320:string, "x = y?"=w318:bool)  [unwired: 8 in, 1 out]
                "ToolStringOut_P1" <- w320
                n145 = call "Auto Inspection_Status.vi"("Action"=enum16{"Initial", "Write", "Read"}."Write", "DataIn"="PROGRAM1", "Station"=Auto_Inspection_Station_Name2."S2Measure", "Data"=Auto_Inspection_Data_Name."CurrentAction", "error in"=w298) -> ()  [unwired: 8 in, 3 out]
                n146 = String Length(string=w320) -> (length=w322:i32)
                n147 = Not(x=w318) -> (.not. x?=w319:bool)
                n148 = Not Equal To 0?(x=w322) -> (x != 0?=w323:bool)
                n149 = Not(x=w323) -> (.not. x?=w321:bool)
                n150 = Or(x=w319, y=w321) -> ()  [unwired: 1 out]
                n151 = call "ToolProgramTest.vi"("error in (no error)"=w315, "VISA resource name"=w314) -> ("Array"=w305:string[])  [unwired: 4 in, 5 out]
                n152 = Index Array(array=w305, index=0) -> (element=w312:string)
                n153 = call "befor_ChkSum.vi"("ToolString Input"=w312) -> ("Array"=w311:string[])  [unwired: 9 in, 1 out]
                n154 = call "Check Sum Test_01.vi"("Array"=w311) -> ("ToolStringOut_01"=w299:string, "x = y?"=w308:bool)  [unwired: 8 in, 1 out]
                "ToolStringOut_P1_2" <- w299
                n155 = global write "Process Global.vi" "S2 Tool String Display"(w299) -> ()
                n156 = String Length(string=w299) -> (length=w309:i32)
                n157 = Not(x=w308) -> (.not. x?=w307:bool)
                n158 = Unbundle By Name(w315) -> ("status"=w303:bool)
                n159 = call "Get ProgReturn Info.vi"("String"=w299) -> ("Chk OK or Fail"=w304:bool)  [unwired: 8 in, 2 out]
                n160 = Not Equal To 0?(x=w309) -> (x != 0?=w310:bool)
                n161 = Not(x=w310) -> (.not. x?=w306:bool)
                n162 = Compound Arithmetic op=OR(invert w304, w307, w306) -> (w302:bool)
                n163 = Or(x=w302, y=w303) -> (x .or. y?=w301:bool)
                n164 = Not(x=w301) -> (.not. x?=w297:bool)
                n165 = Increment(x=w324) -> (x+1=w349:i32)
                n166 = Select(t=w349, s=w301, f=w324) -> (s? t:f=w346:i32)
                n167 = case shown="False" w297 {
                  frame False {
                    n168 = call "Auto Inspection_Status.vi"("Action"=enum16{"Initial", "Write", "Read"}."Write", "DataIn"="PROGRAM1 RETRY", "Station"=Auto_Inspection_Station_Name2."S2Measure", "Data"=Auto_Inspection_Data_Name."ItemSN(TimeCode)") -> ()  [unwired: 9 in, 3 out]
                  }
                  frame True {
                  }
                }
                n169 = Select(t="OK" ("DataIn"), s=w304, f="NG" ("DataIn")) -> (s? t:f=w333:string)
                n170 = Greater Or Equal?(x=w346, y=w348) -> (x >= y?=w347:bool)
                n171 = global read "Main Glb.vi" "Input Registers0-99"() -> (w327:u16[])
                n172 = case shown="False" w347 {
                  tunnel: [errorcluster {"status"=FALSE, "code"=0, "source"=""} ("error constant") errorcluster {"status"=TRUE, "code"=18202, "source"=""} ("error constant")] -> w300
                  tunnel: w346 -> [w379 _]
                  tunnel: [w379 0] -> w325
                  frame False {
                  }
                  frame True {
                  }
                }
                n173 = call "Red PLC InReg.vi"("length"=10, "index"=20, "Input Registers Arr"=w327) -> ("Rad In Reg"=w294:string)  [unwired: 7 in, 1 out]
                n174 = Increment(x=w341) -> (x+1=w350:i32)
                n175 = call "Cub Meaasure FGV.vi"("Action"=Table_Save."Write" ("Enum"), "Save Index"=MeasureDisplayTab."Programe(Tool Programe)", "DataIn"=w333, "SN"=w294) -> ()  [unwired: 8 in, 8 out]
                n176 = Select(t=w350, s=w297, f=w341) -> (s? t:f=w339:i32)
                n177 = global write "Main Glb.vi" "S2 Barcode ID"(w294) -> ()
                n178 = call "Cub Meaasure FGV.vi"("Action"=Table_Save."REad" ("Enum"), "Save Index"=MeasureDisplayTab."Tray Barcode", "SN"=w294) -> ("Read Index Data"=w293:string)  [unwired: 9 in, 7 out]
                n179 = global write "Main Glb.vi" "S2 Tary ID"(w293) -> ()
                n180 = case shown="No Error" w300 {
                  tunnel: w297 -> [w356 _]
                  frame No Error {
                    n181 = case shown="True" w356 {
                      frame False {
                      }
                      frame True {
                        w366 = T5[] [enum."S2站燒入執行_26", enum."S2站燒入OK_27"] items=["S2站PC動作中_20", "電流量測完成產品OK_21", "電流量測完成產品NG_22", "S2站Format 執行_23", "S2 Format OK_24", "S2 Format NG_25", "S2站燒入執行_26", "S2站燒入OK_27", "S2站燒入NG_28", "S2站動作完成_29", "S3 PC動作中_30", "S3 Format 此站執行_31", "S3 Format OK_32", "S3 Format NG_33", "S3 燒入程式 此站執行_34", "S3 燒入程式 OK_35", "S3 燒入程式 NG_36", "S3 備用_37", "S3 備用_38", "S3 動作完成_39", "S4 PC動作中_40", "S4 量測完成 產品正常_41", "S4 量測完成 產品NG_42", "S4 Format 此站執行_43", "S4 Format OK_44", "S4 Format NG_45", "S4 燒入 此站不執行_46", "S4 燒入程式 OK_47", "S4 燒入程式 NG_48", "S4 藍芽Scan OK_49", "S4 藍芽Scan NG_50", "S4 動作完成_51", "給PLC要量電流訊號", "給PLC要量電壓訊號"]
                        n182 = global read "Process Global.vi" "S2Tool Action"() -> (w361:bool[])
                        n183 = call "Set OutputPLC.vi"("Address In"=20, "Array 2"=w366, "Sat Coils"=bool[] [TRUE]) -> ()  [unwired: 7 in, 1 out]
                        n184 = Replace Array Subset(array=w361, new element=TRUE ("new element/subarray"), index=3) -> (w358:bool[])
                        n185 = global write "Process Global.vi" "S2Tool Action"(w358) -> ()
                        n186 = call "Auto Inspection_Status.vi"("Action"=enum16{"Initial", "Write", "Read"}."Write", "DataIn"="PROGRAM1成功", "Station"=Auto_Inspection_Station_Name2."S2Measure", "Data"=Auto_Inspection_Data_Name."ItemSN(TimeCode)") -> ()  [unwired: 9 in, 3 out]
                      }
                    }
                  }
                  frame Error {
                    w378 = T5[] [enum."S2站燒入執行_26", enum."S2站燒入NG_28"] items=["S2站PC動作中_20", "電流量測完成產品OK_21", "電流量測完成產品NG_22", "S2站Format 執行_23", "S2 Format OK_24", "S2 Format NG_25", "S2站燒入執行_26", "S2站燒入OK_27", "S2站燒入NG_28", "S2站動作完成_29", "S3 PC動作中_30", "S3 Format 此站執行_31", "S3 Format OK_32", "S3 Format NG_33", "S3 燒入程式 此站執行_34", "S3 燒入程式 OK_35", "S3 燒入程式 NG_36", "S3 備用_37", "S3 備用_38", "S3 動作完成_39", "S4 PC動作中_40", "S4 量測完成 產品正常_41", "S4 量測完成 產品NG_42", "S4 Format 此站執行_43", "S4 Format OK_44", "S4 Format NG_45", "S4 燒入 此站不執行_46", "S4 燒入程式 OK_47", "S4 燒入程式 NG_48", "S4 藍芽Scan OK_49", "S4 藍芽Scan NG_50", "S4 動作完成_51", "給PLC要量電流訊號", "給PLC要量電壓訊號"]
                    n187 = global read "Process Global.vi" "S2Tool Action"() -> (w372:bool[])
                    n188 = Replace Array Subset(array=w372, new element=FALSE ("new element/subarray"), index=3) -> (w369:bool[])
                    n189 = global write "Process Global.vi" "S2Tool Action"(w369) -> ()
                    n190 = call "Set OutputPLC.vi"("Address In"=20, "Array 2"=w378, "Sat Coils"=bool[] [TRUE]) -> ()  [unwired: 7 in, 1 out]
                    n191 = call "Auto Inspection_Status.vi"("Action"=enum16{"Initial", "Write", "Read"}."Write", "DataIn"="PROGRAM1失敗", "Station"=Auto_Inspection_Station_Name2."S2Measure", "Data"=Auto_Inspection_Data_Name."ItemSN(TimeCode)") -> ()  [unwired: 9 in, 3 out]
                  }
                }
              }
              frame "P2" {
                # "收尋S2站條碼"
                n192 = call "Retry Num.vi"("String"=w394) -> ("Numeric"=w415:i32, "retry次數"=w418:string[])  [unwired: 9 in]
                n193 = call "Auto Inspection_Status.vi"("Action"=enum16{"Initial", "Write", "Read"}."Write", "DataIn"="PROGRAM2", "Station"=Auto_Inspection_Station_Name2."S2Measure", "Data"=Auto_Inspection_Data_Name."CurrentAction", "error in"=w389) -> ()  [unwired: 8 in, 3 out]
                n194 = Index Array(array=w397, index=StationCmdSelect."Command") -> (element=w419:string)
                n195 = local write "retry次數 2"(w418) -> ()
                n196 = local write "CurrentCmd 2"(w419) -> ()
                n197 = call "Tool RS232 test.vi"("error in (no error)"=w389, "Cmd In"=w419, "VISA resource name"=w398) -> ("error out"=w411:errorcluster, "receive string"=→"Program1 receive 2":string)  [unwired: 7 in]
                n198 = local write "Retry 2"(w415) -> ()
                n199 = Unbundle By Name(w411) -> ("status"=w413:bool)
                n200 = Increment(x=w395) -> (x+1=w414:i32)
                n201 = Not(x=w413) -> (.not. x?=w388:bool)
                n202 = Select(t=w414, s=w413, f=w395) -> (s? t:f=w417:i32)
                n203 = Increment(x=w396) -> (x+1=w412:i32)
                n204 = Greater Or Equal?(x=w417, y=w415) -> (x >= y?=w416:bool)
                n205 = case shown="True" w416 {
                  tunnel: [errorcluster {"status"=FALSE, "code"=0, "source"=""} ("error constant") errorcluster {"status"=TRUE, "code"=18202, "source"=""} ("error constant")] -> w390
                  tunnel: w417 -> [w449 _]
                  tunnel: [w449 0] -> w392
                  frame False {
                  }
                  frame True {
                  }
                }
                n206 = Select(t=w412, s=w388, f=w396) -> (s? t:f=w393:i32)
                n207 = case shown="False" w388 {
                  frame False {
                    n208 = call "Auto Inspection_Status.vi"("Action"=enum16{"Initial", "Write", "Read"}."Write", "DataIn"="PROGRAM2 RETRY", "Station"=Auto_Inspection_Station_Name2."S2Measure", "Data"=Auto_Inspection_Data_Name."ItemSN(TimeCode)") -> ()  [unwired: 9 in, 3 out]
                  }
                  frame True {
                  }
                }
                n209 = Select(t="OK" ("DataIn"), s=w388, f="NG" ("DataIn")) -> (s? t:f=w420:string)
                n210 = global read "Main Glb.vi" "Input Registers0-99"() -> (w421:u16[])
                n211 = call "Red PLC InReg.vi"("length"=10, "index"=20, "Input Registers Arr"=w421) -> ("Rad In Reg"=w384:string)  [unwired: 7 in, 1 out]
                n212 = call "Cub Meaasure FGV.vi"("Action"=Table_Save."Write" ("Enum"), "Save Index"=MeasureDisplayTab."Programe(Tool Programe)", "DataIn"=w420, "SN"=w384) -> ("error out"=w385:errorcluster)  [unwired: 8 in, 7 out]
                n213 = global write "Main Glb.vi" "S2 Barcode ID"(w384) -> ()
                n214 = case shown="Error .." w390 {
                  tunnel: w388 -> [w426 _]
                  frame No Error {
                    n215 = case shown="True" w426 {
                      frame False {
                      }
                      frame True {
                        w436 = T5[] [enum."S2站燒入執行_26", enum."S2站燒入OK_27"] items=["S2站PC動作中_20", "電流量測完成產品OK_21", "電流量測完成產品NG_22", "S2站Format 執行_23", "S2 Format OK_24", "S2 Format NG_25", "S2站燒入執行_26", "S2站燒入OK_27", "S2站燒入NG_28", "S2站動作完成_29", "S3 PC動作中_30", "S3 Format 此站執行_31", "S3 Format OK_32", "S3 Format NG_33", "S3 燒入程式 此站執行_34", "S3 燒入程式 OK_35", "S3 燒入程式 NG_36", "S3 備用_37", "S3 備用_38", "S3 動作完成_39", "S4 PC動作中_40", "S4 量測完成 產品正常_41", "S4 量測完成 產品NG_42", "S4 Format 此站執行_43", "S4 Format OK_44", "S4 Format NG_45", "S4 燒入 此站不執行_46", "S4 燒入程式 OK_47", "S4 燒入程式 NG_48", "S4 藍芽Scan OK_49", "S4 藍芽Scan NG_50", "S4 動作完成_51", "給PLC要量電流訊號", "給PLC要量電壓訊號"]
                        n216 = call "Set OutputPLC.vi"("Address In"=20, "Array 2"=w436, "Sat Coils"=bool[] [TRUE]) -> ()  [unwired: 7 in, 1 out]
                        n217 = global read "Process Global.vi" "S2Tool Action"() -> (w431:bool[])
                        n218 = call "Auto Inspection_Status.vi"("Action"=enum16{"Initial", "Write", "Read"}."Write", "DataIn"="PROGRAM2成功", "Station"=Auto_Inspection_Station_Name2."S2Measure", "Data"=Auto_Inspection_Data_Name."ItemSN(TimeCode)") -> ()  [unwired: 9 in, 3 out]
                        n219 = Replace Array Subset(array=w431, new element=TRUE ("new element/subarray"), index=3) -> (w428:bool[])
                        n220 = global write "Process Global.vi" "S2Tool Action"(w428) -> ()
                      }
                    }
                  }
                  frame Error {
                    w448 = T5[] [enum."S2站燒入執行_26", enum."S2站燒入NG_28"] items=["S2站PC動作中_20", "電流量測完成產品OK_21", "電流量測完成產品NG_22", "S2站Format 執行_23", "S2 Format OK_24", "S2 Format NG_25", "S2站燒入執行_26", "S2站燒入OK_27", "S2站燒入NG_28", "S2站動作完成_29", "S3 PC動作中_30", "S3 Format 此站執行_31", "S3 Format OK_32", "S3 Format NG_33", "S3 燒入程式 此站執行_34", "S3 燒入程式 OK_35", "S3 燒入程式 NG_36", "S3 備用_37", "S3 備用_38", "S3 動作完成_39", "S4 PC動作中_40", "S4 量測完成 產品正常_41", "S4 量測完成 產品NG_42", "S4 Format 此站執行_43", "S4 Format OK_44", "S4 Format NG_45", "S4 燒入 此站不執行_46", "S4 燒入程式 OK_47", "S4 燒入程式 NG_48", "S4 藍芽Scan OK_49", "S4 藍芽Scan NG_50", "S4 動作完成_51", "給PLC要量電流訊號", "給PLC要量電壓訊號"]
                    n221 = call "Set OutputPLC.vi"("Address In"=20, "Array 2"=w448, "Sat Coils"=bool[] [TRUE]) -> ()  [unwired: 7 in, 1 out]
                    n222 = global read "Process Global.vi" "S2Tool Action"() -> (w442:bool[])
                    n223 = call "Auto Inspection_Status.vi"("Action"=enum16{"Initial", "Write", "Read"}."Write", "DataIn"="PROGRAM2失敗", "Station"=Auto_Inspection_Station_Name2."S2Measure", "Data"=Auto_Inspection_Data_Name."ItemSN(TimeCode)") -> ()  [unwired: 9 in, 3 out]
                    n224 = Replace Array Subset(array=w442, new element=FALSE ("new element/subarray"), index=3) -> (w439:bool[])
                    n225 = global write "Process Global.vi" "S2Tool Action"(w439) -> ()
                  }
                }
                n226 = call "Cub Meaasure FGV.vi"("Action"=Table_Save."REad" ("Enum"), "Save Index"=MeasureDisplayTab."Tray Barcode", "SN"=w384, "error in (no error)"=w385) -> ("Read Index Data"=w383:string)  [unwired: 8 in, 7 out]
                n227 = global write "Main Glb.vi" "S2 Tary ID"(w383) -> ()
              }
              frame "S1" {
                # "收尋S2站條碼"
                n228 = call "Retry Num.vi"("String"=w493) -> ("Numeric"=w499:i32, "retry次數"=w496:string[])  [unwired: 9 in]
                n229 = Index Array(array=w492, index=StationCmdSelect."Command") -> (element=w491:string)
                n230 = local write "retry次數"(w496) -> ()
                n231 = call "Tool RS232 test.vi"("error in (no error)"=w456, "Cmd In"=w491, "VISA resource name"=w469) -> ("error out"=w502:errorcluster, "receive string"=→"S1 receive":string)  [unwired: 7 in]
                n232 = local write "CurrentCmd"(w491) -> ()
                n233 = call "Auto Inspection_Status.vi"("Action"=enum16{"Initial", "Write", "Read"}."Write", "DataIn"="SCAN1", "Station"=Auto_Inspection_Station_Name2."S2Measure", "Data"=Auto_Inspection_Data_Name."CurrentAction") -> ()  [unwired: 9 in, 3 out]
                n234 = local write "Retry"(w499) -> ()
                n235 = Unbundle By Name(w502) -> ("status"=w489:bool)
                n236 = call "ToolScanTest.vi"("error in (no error)"=w456, "VISA resource name"=refnum<visa-resource-name> "COM10") -> ("error out"=w466:errorcluster, "read string 6"=w462:string, "Array"=w463:string[])  [unwired: 4 in, 3 out]
                "Blue Scan receive" <- w462
                "Array" <- w463
                n237 = String Length(string=w462) -> (length=w461:i32)
                n238 = call <vilib>:"Clear Errors.vi"("error in (no error)"=w466) -> ()  [unwired: 5 in, 2 out]
                n239 = Not Equal?(x=w461, y=0) -> (x != y?=w459:bool)
                n240 = call "Check Sum Test_01.vi"("Array"=w463) -> ("ToolStringOut_01"=w453:string, "ChkSum"=→"S1 ChkSum":string, "x = y?"=w465:bool)  [unwired: 8 in]
                "S1 ToolStringOut" <- w453
                n241 = Not(x=w459) -> (.not. x?=w458:bool)
                n242 = Not(x=w465) -> (.not. x?=w457:bool)
                n243 = Or(x=w457, y=w458) -> (x .or. y?=w455:bool)
                n244 = global write "Process Global.vi" "S2 Tool String Display"(w453) -> ()
                n245 = Or(x=w455, y=w489) -> (x .or. y?=w488:bool)
                n246 = Not(x=w488) -> (.not. x?=w454:bool)
                n247 = Increment(x=w470) -> (x+1=w500:i32)
                n248 = Select(t=w500, s=w488, f=w470) -> (s? t:f=w497:i32)
                n249 = Increment(x=w468) -> (x+1=w501:i32)
                n250 = Greater Or Equal?(x=w497, y=w499) -> (x >= y?=w498:bool)
                n251 = Select(t=w501, s=w454, f=w468) -> (s? t:f=w494:i32)
                n252 = global read "Main Glb.vi" "Input Registers0-99"() -> (w473:u16[])
                n253 = Select(t="OK" ("DataIn"), s=w454, f="NG" ("DataIn")) -> (s? t:f=w480:string)
                n254 = disable-structure shown="Disabled" {
                  disable-tunnel: [w505 _] -> w487
                  disable-tunnel: w454 -> [w504 _]
                  frame Disabled {
                    n255 = case shown="True" w504 {
                      tunnel: [w506 w510] -> w505
                      frame False {
                        w508 = T5[] [enum."S4 量測完成 產品NG_42"] items=["S2站PC動作中_20", "電流量測完成產品OK_21", "電流量測完成產品NG_22", "S2站Format 執行_23", "S2 Format OK_24", "S2 Format NG_25", "S2站燒入執行_26", "S2站燒入OK_27", "S2站燒入NG_28", "S2站動作完成_29", "S3 PC動作中_30", "S3 Format 此站執行_31", "S3 Format OK_32", "S3 Format NG_33", "S3 燒入程式 此站執行_34", "S3 燒入程式 OK_35", "S3 燒入程式 NG_36", "S3 備用_37", "S3 備用_38", "S3 動作完成_39", "S4 PC動作中_40", "S4 量測完成 產品正常_41", "S4 量測完成 產品NG_42", "S4 Format 此站執行_43", "S4 Format OK_44", "S4 Format NG_45", "S4 燒入 此站不執行_46", "S4 燒入程式 OK_47", "S4 燒入程式 NG_48", "S4 藍芽Scan OK_49", "S4 藍芽Scan NG_50", "S4 動作完成_51", "給PLC要量電流訊號", "給PLC要量電壓訊號"]
                        n256 = call "Set OutputPLC.vi"("Array"=w508, "Address In"=20) -> ("Error Out"=w506:errorcluster[])  [unwired: 9 in]
                      }
                      frame True {
                        w509 = T5[] [enum."S4 量測完成 產品正常_41"] items=["S2站PC動作中_20", "電流量測完成產品OK_21", "電流量測完成產品NG_22", "S2站Format 執行_23", "S2 Format OK_24", "S2 Format NG_25", "S2站燒入執行_26", "S2站燒入OK_27", "S2站燒入NG_28", "S2站動作完成_29", "S3 PC動作中_30", "S3 Format 此站執行_31", "S3 Format OK_32", "S3 Format NG_33", "S3 燒入程式 此站執行_34", "S3 燒入程式 OK_35", "S3 燒入程式 NG_36", "S3 備用_37", "S3 備用_38", "S3 動作完成_39", "S4 PC動作中_40", "S4 量測完成 產品正常_41", "S4 量測完成 產品NG_42", "S4 Format 此站執行_43", "S4 Format OK_44", "S4 Format NG_45", "S4 燒入 此站不執行_46", "S4 燒入程式 OK_47", "S4 燒入程式 NG_48", "S4 藍芽Scan OK_49", "S4 藍芽Scan NG_50", "S4 動作完成_51", "給PLC要量電流訊號", "給PLC要量電壓訊號"]
                        n257 = call "Set OutputPLC.vi"("Array"=w509, "Address In"=20) -> ("Error Out"=w510:errorcluster[])  [unwired: 9 in]
                      }
                    }
                  }
                  frame Enabled {
                  }
                }
                n258 = call "Red PLC InReg.vi"("length"=10, "index"=20, "Input Registers Arr"=w473) -> ("Rad In Reg"=w474:string)  [unwired: 7 in, 1 out]
                n259 = call "Cub Meaasure FGV.vi"("Action"=Table_Save."Write" ("Enum"), "Save Index"=MeasureDisplayTab."FSKscanl_315(FSK scan)", "DataIn"=w480, "SN"=w474) -> ()  [unwired: 8 in, 8 out]
                n260 = case shown="False" w498 {
                  tunnel: [errorcluster {"status"=FALSE, "code"=0, "source"=""} ("error constant") errorcluster {"status"=TRUE, "code"=18203, "source"=""} ("error constant")] -> w486
                  tunnel: w497 -> [w512 _]
                  tunnel: [w512 0] -> w471
                  frame False {
                  }
                  frame True {
                  }
                }
                n261 = Merge Errors(w487, w486) -> (w485:errorcluster)
              }
              frame "S2" {
                # "收尋S2站條碼"
                n262 = call "Retry Num.vi"("String"=w537) -> ("Numeric"=w554:i32, "retry次數"=w551:string[])  [unwired: 9 in]
                n263 = Index Array(array=w538, index=StationCmdSelect."Command") -> (element=w550:string)
                n264 = call "ToolScanTest.vi"("error in (no error)"=w539, "VISA resource name"=refnum<visa-resource-name> "COM10") -> ("error out"=w549:errorcluster, "read string 3"=w547:string)  [unwired: 4 in, 4 out]
                "Blue Scan2 receive" <- w547
                n265 = local write "retry次數"(w551) -> ()
                n266 = call "Tool RS232 test.vi"("error in (no error)"=w539, "Cmd In"=w550, "VISA resource name"=w516) -> ("error out"=w557:errorcluster, "receive string"=→"S2 receive":string)  [unwired: 7 in]
                n267 = local write "CurrentCmd"(w550) -> ()
                n268 = call <vilib>:"Clear Errors.vi"("error in (no error)"=w549) -> ()  [unwired: 5 in, 2 out]
                n269 = local write "Retry"(w554) -> ()
                n270 = Unbundle By Name(w557) -> ("status"=w544:bool)
                n271 = String Length(string=w547) -> (length=w548:i32)
                n272 = Not Equal To 0?(x=w548) -> (x != 0?=w546:bool)
                n273 = Not(x=w546) -> (.not. x?=w545:bool)
                n274 = Or(x=w545, y=w544) -> (x .or. y?=w543:bool)
                n275 = Not(x=w543) -> (.not. x?=w520:bool)
                n276 = Increment(x=w517) -> (x+1=w555:i32)
                n277 = Select(t=w555, s=w543, f=w517) -> (s? t:f=w552:i32)
                n278 = Increment(x=w540) -> (x+1=w556:i32)
                n279 = Greater Or Equal?(x=w552, y=w554) -> (x >= y?=w553:bool)
                n280 = Select(t=w556, s=w520, f=w540) -> (s? t:f=w536:i32)
                n281 = call "Auto Inspection_Status.vi"("Action"=enum16{"Initial", "Write", "Read"}."Write", "DataIn"="SCAN2", "Station"=Auto_Inspection_Station_Name2."S2Measure", "Data"=Auto_Inspection_Data_Name."CurrentAction") -> ()  [unwired: 9 in, 3 out]
                n282 = disable-structure shown="Disabled" {
                  disable-tunnel: [w561 _] -> w535
                  disable-tunnel: w520 -> [w560 _]
                  frame Disabled {
                    n283 = case shown="True" w560 {
                      tunnel: [w562 w566] -> w561
                      frame False {
                        w564 = T5[] [enum."S4 量測完成 產品NG_42"] items=["S2站PC動作中_20", "電流量測完成產品OK_21", "電流量測完成產品NG_22", "S2站Format 執行_23", "S2 Format OK_24", "S2 Format NG_25", "S2站燒入執行_26", "S2站燒入OK_27", "S2站燒入NG_28", "S2站動作完成_29", "S3 PC動作中_30", "S3 Format 此站執行_31", "S3 Format OK_32", "S3 Format NG_33", "S3 燒入程式 此站執行_34", "S3 燒入程式 OK_35", "S3 燒入程式 NG_36", "S3 備用_37", "S3 備用_38", "S3 動作完成_39", "S4 PC動作中_40", "S4 量測完成 產品正常_41", "S4 量測完成 產品NG_42", "S4 Format 此站執行_43", "S4 Format OK_44", "S4 Format NG_45", "S4 燒入 此站不執行_46", "S4 燒入程式 OK_47", "S4 燒入程式 NG_48", "S4 藍芽Scan OK_49", "S4 藍芽Scan NG_50", "S4 動作完成_51", "給PLC要量電流訊號", "給PLC要量電壓訊號"]
                        n284 = call "Set OutputPLC.vi"("Array"=w564, "Address In"=20) -> ("Error Out"=w562:errorcluster[])  [unwired: 9 in]
                      }
                      frame True {
                        w565 = T5[] [enum."S4 量測完成 產品正常_41"] items=["S2站PC動作中_20", "電流量測完成產品OK_21", "電流量測完成產品NG_22", "S2站Format 執行_23", "S2 Format OK_24", "S2 Format NG_25", "S2站燒入執行_26", "S2站燒入OK_27", "S2站燒入NG_28", "S2站動作完成_29", "S3 PC動作中_30", "S3 Format 此站執行_31", "S3 Format OK_32", "S3 Format NG_33", "S3 燒入程式 此站執行_34", "S3 燒入程式 OK_35", "S3 燒入程式 NG_36", "S3 備用_37", "S3 備用_38", "S3 動作完成_39", "S4 PC動作中_40", "S4 量測完成 產品正常_41", "S4 量測完成 產品NG_42", "S4 Format 此站執行_43", "S4 Format OK_44", "S4 Format NG_45", "S4 燒入 此站不執行_46", "S4 燒入程式 OK_47", "S4 燒入程式 NG_48", "S4 藍芽Scan OK_49", "S4 藍芽Scan NG_50", "S4 動作完成_51", "給PLC要量電流訊號", "給PLC要量電壓訊號"]
                        n285 = call "Set OutputPLC.vi"("Array"=w565, "Address In"=20) -> ("Error Out"=w566:errorcluster[])  [unwired: 9 in]
                      }
                    }
                  }
                  frame Enabled {
                  }
                }
                n286 = case shown="False" w553 {
                  tunnel: [errorcluster {"status"=FALSE, "code"=0, "source"=""} ("error constant") errorcluster {"status"=TRUE, "code"=18204, "source"=""} ("error constant")] -> w534
                  tunnel: w552 -> [w568 _]
                  tunnel: [w568 0] -> w518
                  frame False {
                  }
                  frame True {
                  }
                }
                n287 = Merge Errors(w535, w534) -> (w533:errorcluster)
                n288 = Select(t="OK" ("DataIn"), s=w520, f="NG" ("DataIn")) -> (s? t:f=w528:string)
                n289 = global read "Main Glb.vi" "Input Registers0-99"() -> (w521:u16[])
                n290 = call "Red PLC InReg.vi"("length"=10, "index"=20, "Input Registers Arr"=w521) -> ("Rad In Reg"=w522:string)  [unwired: 7 in, 1 out]
                n291 = call "Cub Meaasure FGV.vi"("Action"=Table_Save."Write" ("Enum"), "Save Index"=MeasureDisplayTab."ASKscan_433(ASK scan)", "DataIn"=w528, "SN"=w522) -> ()  [unwired: 8 in, 8 out]
              }
              frame "D" {
                n292 = Index Array(array=w583) -> (element=w582:i32)  [unwired: 1 in]
                n293 = Multiply(x=1000, y=w582) -> (x*y=w581:i32)
                n294 = Wait (ms)(milliseconds to wait=w581) -> ()  [unwired: 1 out]
                n295 = Increment(x=w578) -> (x+1=w577:i32)
                n296 = call "Auto Inspection_Status.vi"("Action"=enum16{"Initial", "Write", "Read"}."Write", "DataIn"="Delay", "Station"=Auto_Inspection_Station_Name2."S2Measure", "Data"=Auto_Inspection_Data_Name."CurrentAction") -> ()  [unwired: 9 in, 3 out]
              }
              frame "T1" {
                w592 = T5[] [enum."給PLC要量電流訊號"] items=["S2站PC動作中_20", "電流量測完成產品OK_21", "電流量測完成產品NG_22", "S2站Format 執行_23", "S2 Format OK_24", "S2 Format NG_25", "S2站燒入執行_26", "S2站燒入OK_27", "S2站燒入NG_28", "S2站動作完成_29", "S3 PC動作中_30", "S3 Format 此站執行_31", "S3 Format OK_32", "S3 Format NG_33", "S3 燒入程式 此站執行_34", "S3 燒入程式 OK_35", "S3 燒入程式 NG_36", "S3 備用_37", "S3 備用_38", "S3 動作完成_39", "S4 PC動作中_40", "S4 量測完成 產品正常_41", "S4 量測完成 產品NG_42", "S4 Format 此站執行_43", "S4 Format OK_44", "S4 Format NG_45", "S4 燒入 此站不執行_46", "S4 燒入程式 OK_47", "S4 燒入程式 NG_48", "S4 藍芽Scan OK_49", "S4 藍芽Scan NG_50", "S4 動作完成_51", "給PLC要量電流訊號", "給PLC要量電壓訊號"]
                n297 = flat-sequence {
                  tunnel: [w602] -> w593
                  tunnel: w590 -> [w601]
                  tunnel: [w601] -> w586
                  frame #0 {
                    n298 = global read "Main Glb.vi" "Discrete Inputs"() -> (w604:bool[])
                    n299 = Index Array(array=w604, index=S2_Station_Input."21_PLC下達可測電流訊號" ("Enum")) -> (element=w602:bool)
                  }
                }
                n300 = call "ModbusCmdIn.vi"("data"=T2 {"starting address"=0, "number of inputs"=0, "Sat Coils"=[], "Holding Registers"=[]}, "Enum"=ModbusCmd."Fetch Discrete Inputs") -> ("error out"=w587:errorcluster)  [unwired: 9 in]
                n301 = call "Set OutputPLC.vi"("Address In"=20, "Array 2"=w592, "Sat Coils"=bool[] [TRUE], "error in (no error)"=w587) -> ("Error Out"=w590:errorcluster[])  [unwired: 6 in]
                n302 = case shown="True" w593 {
                  tunnel: w599 -> [_ w654]
                  tunnel: w598 -> [w608 w652]
                  tunnel: [w608 w650] -> w597
                  tunnel: [errorcluster {"status"=FALSE, "code"=0, "source"=""} ("error IO") w610] -> w596
                  tunnel: [0 ("Err Count") w611] -> w595
                  tunnel: w594 -> [_ w634]
                  tunnel: w586 -> [_ w625]
                  frame False {
                    n303 = Wait (ms)(milliseconds to wait=u32 400) -> ()  [unwired: 1 out]
                  }
                  frame True {
                    w658 = u16 3 items=["SYSTem:VERSion?", "SYSTem:ERRor?", "*IDN?", "MEAS:CURR:DC?", "MEAS:VOLT?", "SYSTem:ERRor?"] ("Ringfor34450A")
                    w657 = u16 5 items=["SYSTem:VERSion?", "SYSTem:ERRor?", "*IDN?", "MEAS:CURR:DC?", "MEAS:VOLT?", "MEAS:VOLT:DC?"] ("RingforIT8511")
                    w655 = u16 1 items=["IT8511", "34450A", "WRBuff"] ("ChangeStatus")
                    # "讀取S2站條碼"
                    # "T1 34450A"
                    # "量電流"
                    n304 = Merge Errors(w625) -> (w627:errorcluster)
                    n305 = call "Retry Num.vi"("String"=w654) -> ("Numeric"=w660:i32, "retry次數"=w659:string[])  [unwired: 9 in]
                    n306 = Merge Errors(w625) -> (w624:errorcluster)
                    n307 = call "Auto Inspection_Status.vi"("Action"=enum16{"Initial", "Write", "Read"}."Write", "DataIn"="34450A儀器測量中", "Station"=Auto_Inspection_Station_Name2."S2Measure", "Data"=Auto_Inspection_Data_Name."CurrentAction", "error in"=w627) -> ()  [unwired: 8 in, 3 out]
                    n308 = local write "retry次數"(w659) -> ()
                    n309 = for {
                      N: 3 -> [_]
                      tunnel: w658 -> [w673]
                      tunnel: w657 -> [w672]
                      tunnel: refnum<visa-resource-name> "USB0::0x2A8D::0xB318::MY59430005::INSTR" ("VISA resource name") -> [w671]
                      tunnel: w655 -> [w670]
                      tunnel: [w669] -> w633
                      tunnel: [w668] -> w628
                      tunnel: [w666] -> w623
                      tunnel: w624 -> [w667]
                      tunnel: [w665] -> w622
                      stop <- w664 continue-if-true
                      n310 = call "MTool34450A.vi"("error in (no error)"=w667, "Ringfor34450A"=w673, "RingforIT8511"=w672, "VISA resource name"=w671, "ChangeStatus"=w670) -> ("error out"=w665:errorcluster, 1:"μA"=w666:string, 2:"μA"=w668:dbl, "read buffer"=w669:string)  [unwired: 3 in]
                      n311 = Unbundle By Name(w665) -> ("status"=w664:bool)
                      n312 = Wait (ms)(milliseconds to wait=u32 100) -> ()  [unwired: 1 out]
                    }
                    "T1 buffer" <- w633
                    "T1 μA" <- w628
                    n313 = local write "Retry"(w660) -> ()
                    n314 = call "ProjectSearchDataName.vi"("element"="$ForceSetBinChk_") -> ("variant"=w630:variant)  [unwired: 7 in, 3 out]
                    n315 = Variant To Data(type=FALSE, Variant=w630) -> (data=w629:bool)  [unwired: 1 in, 1 out]
                    n316 = Unbundle By Name(w622) -> ("status"=w651:bool)
                    n317 = Increment(x=w634) -> (x+1=w661:i32)
                    n318 = global write "Process Global.vi" "T1 Current00"(w628) -> ()
                    n319 = Select(t=w661, s=w651, f=w634) -> (s? t:f=w653:i32)
                    n320 = Greater Or Equal?(x=w653, y=w660) -> (x >= y?=w649:bool)
                    n321 = call "LineScan量測值轉換.vi"("位數"=4, "error in (no error)"=w622, "input string"=w633, "PLC address"=20) -> ("error out"=w620:errorcluster)  [unwired: 6 in, 1 out]
                    n322 = Not(x=w651) -> (.not. x?=w626:bool)
                    n323 = case shown="True" w629 {
                      tunnel: w628 -> [w681 w690]
                      tunnel: [w682 w689] -> w614
                      tunnel: w626 -> [w682 _]
                      tunnel: w622 -> [_ w686]
                      tunnel: [errorcluster {"status"=FALSE, "code"=0, "source"=""} ("error IO") w683] -> w621
                      frame False {
                        n324 = Number To Fractional String(number=w681) -> (F-format string=w679:string)  [unwired: 3 in]
                        n325 = String Subset(string=w679, length (rest)=5 ("length (rest)")) -> ()  [unwired: 1 in, 1 out]
                      }
                      frame True {
                        n326 = call "ProjectSearchDataName.vi"("error in (no error)"=w686, "element"="$Current Up") -> ("error out"=w685:errorcluster, "variant"=w695:variant)  [unwired: 6 in, 2 out]
                        n327 = call "ProjectSearchDataName.vi"("error in (no error)"=w686, "element"="$Current Dn") -> ("error out"=w684:errorcluster, "variant"=w694:variant)  [unwired: 6 in, 2 out]
                        n328 = Variant To Data(type=0.0, Variant=w695) -> (data=w692:dbl)  [unwired: 1 in, 1 out]
                        n329 = Variant To Data(type=0.0, Variant=w694) -> (data=w691:dbl)  [unwired: 1 in, 1 out]
                        n330 = Merge Errors(w685, w684) -> (w683:errorcluster)
                        n331 = In Range and Coerce(upper limit=w692, x=w690, lower limit=w691) -> (In Range?=w689:bool)  [unwired: 1 out]
                      }
                    }
                    n332 = case shown="False" w649 {
                      tunnel: [errorcluster {"status"=FALSE, "code"=0, "source"=""} ("error constant") errorcluster {"status"=TRUE, "code"=18205, "source"=""} ("error constant")] -> w610
                      tunnel: w653 -> [w737 _]
                      tunnel: [w737 0] -> w613
                      frame False {
                      }
                      frame True {
                      }
                    }
                    n333 = Increment(x=w652) -> (x+1=w662:i32)
                    n334 = Merge Errors(w621, w620) -> (w619:errorcluster)
                    n335 = Select(t=w662, s=w614, f=w652) -> (s? t:f=w650:i32)
                    n336 = Select(t=w623, s=w614, f="NG" ("DataIn")) -> (s? t:f=w642:string)
                    n337 = global read "Main Glb.vi" "Input Registers0-99"() -> (w636:u16[])
                    n338 = Merge Errors(w619) -> (w617:errorcluster)
                    n339 = case shown="False" w626 {
                      frame False {
                        n340 = call "Auto Inspection_Status.vi"("Action"=enum16{"Initial", "Write", "Read"}."Write", "DataIn"="T1 RETRY", "Station"=Auto_Inspection_Station_Name2."S2Measure", "Data"=Auto_Inspection_Data_Name."ItemSN(TimeCode)") -> ()  [unwired: 9 in, 3 out]
                      }
                      frame True {
                      }
                    }
                    n341 = call "wait.vi"("error in"=w617, "wait(ms)"=u32 100) -> ("error out"=w616:errorcluster)  [unwired: 9 in]
                    n342 = Increment(x=w613) -> (x+1=w612:i32)
                    n343 = call "Red PLC InReg.vi"("error in (no error)"=w616, "length"=10, "index"=20, "Input Registers Arr"=w636) -> ("error out"=w618:errorcluster, "Rad In Reg"=w637:string)  [unwired: 6 in]
                    n344 = Select(t=w613, s=w614, f=w612) -> (s? t:f=w611:i32)
                    n345 = call "Cub Meaasure FGV.vi"("Action"=Table_Save."Write" ("Enum"), "Save Index"=MeasureDisplayTab."耗電流 uA(電流表)", "DataIn"=w642, "SN"=w637, "error in (no error)"=w618) -> ()  [unwired: 7 in, 8 out]
                    n346 = case shown="Error .." w610 {
                      selector: w610 -> [w697 _]
                      tunnel: w614 -> [w698 _]
                      frame No Error {
                        n347 = case shown="True" w698 {
                          tunnel: [w699 w708] -> _
                          tunnel: w697 -> [w700 w702]
                          frame False {
                            n348 = Build Array(w700) -> (w699:errorcluster[])
                          }
                          frame True {
                            w709 = T5[] [enum."給PLC要量電流訊號"] items=["S2站PC動作中_20", "電流量測完成產品OK_21", "電流量測完成產品NG_22", "S2站Format 執行_23", "S2 Format OK_24", "S2 Format NG_25", "S2站燒入執行_26", "S2站燒入OK_27", "S2站燒入NG_28", "S2站動作完成_29", "S3 PC動作中_30", "S3 Format 此站執行_31", "S3 Format OK_32", "S3 Format NG_33", "S3 燒入程式 此站執行_34", "S3 燒入程式 OK_35", "S3 燒入程式 NG_36", "S3 備用_37", "S3 備用_38", "S3 動作完成_39", "S4 PC動作中_40", "S4 量測完成 產品正常_41", "S4 量測完成 產品NG_42", "S4 Format 此站執行_43", "S4 Format OK_44", "S4 Format NG_45", "S4 燒入 此站不執行_46", "S4 燒入程式 OK_47", "S4 燒入程式 NG_48", "S4 藍芽Scan OK_49", "S4 藍芽Scan NG_50", "S4 動作完成_51", "給PLC要量電流訊號", "給PLC要量電壓訊號"]
                            w717 = T5[] [enum."電流量測完成產品OK_21"] items=["S2站PC動作中_20", "電流量測完成產品OK_21", "電流量測完成產品NG_22", "S2站Format 執行_23", "S2 Format OK_24", "S2 Format NG_25", "S2站燒入執行_26", "S2站燒入OK_27", "S2站燒入NG_28", "S2站動作完成_29", "S3 PC動作中_30", "S3 Format 此站執行_31", "S3 Format OK_32", "S3 Format NG_33", "S3 燒入程式 此站執行_34", "S3 燒入程式 OK_35", "S3 燒入程式 NG_36", "S3 備用_37", "S3 備用_38", "S3 動作完成_39", "S4 PC動作中_40", "S4 量測完成 產品正常_41", "S4 量測完成 產品NG_42", "S4 Format 此站執行_43", "S4 Format OK_44", "S4 Format NG_45", "S4 燒入 此站不執行_46", "S4 燒入程式 OK_47", "S4 燒入程式 NG_48", "S4 藍芽Scan OK_49", "S4 藍芽Scan NG_50", "S4 動作完成_51", "給PLC要量電流訊號", "給PLC要量電壓訊號"]
                            n349 = global read "Process Global.vi" "S2Tool Action"() -> (w716:bool[])
                            n350 = Replace Array Subset(array=w716, new element=TRUE ("new element/subarray"), index=5) -> (w703:bool[])
                            n351 = global write "Process Global.vi" "S2Tool Action"(w703) -> ()
                            n352 = call "Set OutputPLC.vi"("Address In"=20, "Array 2"=w717, "Sat Coils"=bool[] [TRUE], "error in (no error)"=w702) -> ("Error Out"=w710:errorcluster[])  [unwired: 6 in]
                            n353 = Merge Errors(w710) -> (w713:errorcluster)
                            n354 = call "Auto Inspection_Status.vi"("Action"=enum16{"Initial", "Write", "Read"}."Write", "DataIn"="T1電流量測完成", "Station"=Auto_Inspection_Station_Name2."S2Measure", "Data"=Auto_Inspection_Data_Name."ItemSN(TimeCode)") -> ()  [unwired: 9 in, 3 out]
                            n355 = call "Set OutputPLC.vi"("Address In"=20, "Array 2"=w709, "Sat Coils"=bool[] [FALSE], "error in (no error)"=w713) -> ("Error Out"=w708:errorcluster[])  [unwired: 6 in]
                          }
                        }
                      }
                      frame Error {
                        (unwired) errorcluster[] [] ("Error Out")
                        (unwired) T5[] [enum."電流量測完成產品NG_22"] items=["S2站PC動作中_20", "電流量測完成產品OK_21", "電流量測完成產品NG_22", "S2站Format 執行_23", "S2 Format OK_24", "S2 Format NG_25", "S2站燒入執行_26", "S2站燒入OK_27", "S2站燒入NG_28", "S2站動作完成_29", "S3 PC動作中_30", "S3 Format 此站執行_31", "S3 Format OK_32", "S3 Format NG_33", "S3 燒入程式 此站執行_34", "S3 燒入程式 OK_35", "S3 燒入程式 NG_36", "S3 備用_37", "S3 備用_38", "S3 動作完成_39", "S4 PC動作中_40", "S4 量測完成 產品正常_41", "S4 量測完成 產品NG_42", "S4 Format 此站執行_43", "S4 Format OK_44", "S4 Format NG_45", "S4 燒入 此站不執行_46", "S4 燒入程式 OK_47", "S4 燒入程式 NG_48", "S4 藍芽Scan OK_49", "S4 藍芽Scan NG_50", "S4 動作完成_51", "給PLC要量電流訊號", "給PLC要量電壓訊號"]
                        w723 = T5[] [enum."給PLC要量電流訊號"] items=["S2站PC動作中_20", "電流量測完成產品OK_21", "電流量測完成產品NG_22", "S2站Format 執行_23", "S2 Format OK_24", "S2 Format NG_25", "S2站燒入執行_26", "S2站燒入OK_27", "S2站燒入NG_28", "S2站動作完成_29", "S3 PC動作中_30", "S3 Format 此站執行_31", "S3 Format OK_32", "S3 Format NG_33", "S3 燒入程式 此站執行_34", "S3 燒入程式 OK_35", "S3 燒入程式 NG_36", "S3 備用_37", "S3 備用_38", "S3 動作完成_39", "S4 PC動作中_40", "S4 量測完成 產品正常_41", "S4 量測完成 產品NG_42", "S4 Format 此站執行_43", "S4 Format OK_44", "S4 Format NG_45", "S4 燒入 此站不執行_46", "S4 燒入程式 OK_47", "S4 燒入程式 NG_48", "S4 藍芽Scan OK_49", "S4 藍芽Scan NG_50", "S4 動作完成_51", "給PLC要量電流訊號", "給PLC要量電壓訊號"]
                        w735 = T5[] [enum."電流量測完成產品NG_22"] items=["S2站PC動作中_20", "電流量測完成產品OK_21", "電流量測完成產品NG_22", "S2站Format 執行_23", "S2 Format OK_24", "S2 Format NG_25", "S2站燒入執行_26", "S2站燒入OK_27", "S2站燒入NG_28", "S2站動作完成_29", "S3 PC動作中_30", "S3 Format 此站執行_31", "S3 Format OK_32", "S3 Format NG_33", "S3 燒入程式 此站執行_34", "S3 燒入程式 OK_35", "S3 燒入程式 NG_36", "S3 備用_37", "S3 備用_38", "S3 動作完成_39", "S4 PC動作中_40", "S4 量測完成 產品正常_41", "S4 量測完成 產品NG_42", "S4 Format 此站執行_43", "S4 Format OK_44", "S4 Format NG_45", "S4 燒入 此站不執行_46", "S4 燒入程式 OK_47", "S4 燒入程式 NG_48", "S4 藍芽Scan OK_49", "S4 藍芽Scan NG_50", "S4 動作完成_51", "給PLC要量電流訊號", "給PLC要量電壓訊號"]
                        n356 = global read "Process Global.vi" "S2Tool Action"() -> (w728:bool[])
                        n357 = Replace Array Subset(array=w728, new element=FALSE ("new element/subarray"), index=5) -> (w725:bool[])
                        n358 = global write "Process Global.vi" "S2Tool Action"(w725) -> ()
                        n359 = call "Set OutputPLC.vi"("Address In"=20, "Array 2"=w735, "Sat Coils"=bool[] [TRUE]) -> ("Error Out"=w721:errorcluster[])  [unwired: 7 in]
                        n360 = call "Auto Inspection_Status.vi"("Action"=enum16{"Initial", "Write", "Read"}."Write", "DataIn"="T1電流量測NG", "Station"=Auto_Inspection_Station_Name2."S2Measure", "Data"=Auto_Inspection_Data_Name."ItemSN(TimeCode)") -> ()  [unwired: 9 in, 3 out]
                        n361 = Merge Errors(w721) -> (w720:errorcluster)
                        n362 = call "Set OutputPLC.vi"("Address In"=20, "Array 2"=w723, "Sat Coils"=bool[] [FALSE], "error in (no error)"=w720) -> ("Error Out"=w719:errorcluster[])  [unwired: 6 in]
                        n363 = for {
                          tunnel: w719 -> [w736] mode=indexing
                          n364 = call <vilib>:"Clear Errors.vi"("error in (no error)"=w736) -> ()  [unwired: 5 in, 2 out]
                        }
                      }
                    }
                  }
                }
              }
              frame "T2" {
                w748 = T5[] [enum."給PLC要量電壓訊號"] items=["S2站PC動作中_20", "電流量測完成產品OK_21", "電流量測完成產品NG_22", "S2站Format 執行_23", "S2 Format OK_24", "S2 Format NG_25", "S2站燒入執行_26", "S2站燒入OK_27", "S2站燒入NG_28", "S2站動作完成_29", "S3 PC動作中_30", "S3 Format 此站執行_31", "S3 Format OK_32", "S3 Format NG_33", "S3 燒入程式 此站執行_34", "S3 燒入程式 OK_35", "S3 燒入程式 NG_36", "S3 備用_37", "S3 備用_38", "S3 動作完成_39", "S4 PC動作中_40", "S4 量測完成 產品正常_41", "S4 量測完成 產品NG_42", "S4 Format 此站執行_43", "S4 Format OK_44", "S4 Format NG_45", "S4 燒入 此站不執行_46", "S4 燒入程式 OK_47", "S4 燒入程式 NG_48", "S4 藍芽Scan OK_49", "S4 藍芽Scan NG_50", "S4 動作完成_51", "給PLC要量電流訊號", "給PLC要量電壓訊號"]
                n365 = flat-sequence {
                  tunnel: [w758] -> w746
                  tunnel: w749 -> [w757]
                  tunnel: [w757] -> w743
                  frame #0 {
                    n366 = global read "Main Glb.vi" "Discrete Inputs"() -> (w760:bool[])
                    n367 = Index Array(array=w760, index=S2_Station_Input."22_PLC下達可測電壓訊號" ("Enum")) -> (element=w758:bool)
                  }
                }
                n368 = call "ModbusCmdIn.vi"("data"=T2 {"starting address"=0, "number of inputs"=0, "Sat Coils"=[FALSE], "Holding Registers"=[]}, "Enum"=ModbusCmd."Fetch Discrete Inputs") -> ("error out"=w744:errorcluster)  [unwired: 9 in]
                n369 = call "Set OutputPLC.vi"("Address In"=20, "Array 2"=w748, "Sat Coils"=bool[] [TRUE], "error in (no error)"=w744) -> ("Error Out"=w749:errorcluster[])  [unwired: 6 in]
                n370 = case shown="True" w746 {
                  tunnel: w755 -> [w764 w801]
                  tunnel: [w764 w800] -> w754
                  tunnel: w753 -> [_ w799]
                  tunnel: [errorcluster {"status"=FALSE, "code"=0, "source"=""} ("error IO") w779] -> w752
                  tunnel: w751 -> [_ w778]
                  tunnel: [0 w777] -> w750
                  tunnel: w743 -> [_ w768]
                  frame False {
                    n371 = Wait (ms)(milliseconds to wait=u32 400) -> ()  [unwired: 1 out]
                  }
                  frame True {
                    w805 = u16 3 items=["SYSTem:VERSion?", "SYSTem:ERRor?", "*IDN?", "MEAS:CURR:DC?", "MEAS:VOLT?", "SYSTem:ERRor?"] ("Ringfor34450A")
                    w804 = u16 5 items=["SYSTem:VERSion?", "SYSTem:ERRor?", "*IDN?", "MEAS:CURR:DC?", "MEAS:VOLT?", "MEAS:VOLT:DC?"] ("RingforIT8511")
                    w802 = u16 0 items=["IT8511", "34450A", "WRBuff"] ("ChangeStatus")
                    # "收尋S2站條碼"
                    # "量電壓"
                    # "T2  T8511A/COM11"
                    n372 = call "Retry Num.vi"("String"=w799) -> ("Numeric"=w811:i32, "retry次數"=w810:string[])  [unwired: 9 in]
                    n373 = Merge Errors(w768) -> (w767:errorcluster)
                    n374 = local write "retry次數"(w810) -> ()
                    n375 = call "Auto Inspection_Status.vi"("Action"=enum16{"Initial", "Write", "Read"}."Write", "DataIn"="儀器測量中", "Station"=Auto_Inspection_Station_Name2."S2Measure", "Data"=Auto_Inspection_Data_Name."CurrentAction", "error in"=w767) -> ()  [unwired: 8 in, 3 out]
                    n376 = local write "Retry"(w811) -> ()
                    n377 = call "MTool34450A.vi"("Ringfor34450A"=w805, "RingforIT8511"=w804, "VISA resource name"=refnum<visa-resource-name> "COM11", "ChangeStatus"=w802) -> ("error out"=w806:errorcluster, "μA"=w772:dbl, "read buffer"=w769:string)  [unwired: 4 in, 1 out]
                    "T2 buffer" <- w769
                    "T2 μA" <- w772
                    n378 = Unbundle By Name(w806) -> ("status"=w808:bool)
                    n379 = call "ProjectSearchDataName.vi"("element"="$ForceSetBinChk_") -> ("variant"=w776:variant)  [unwired: 7 in, 3 out]
                    n380 = global write "Process Global.vi" "T2 Voltage"(w769) -> ()
                    n381 = Variant To Data(type=FALSE, Variant=w776) -> (data=w773:bool)  [unwired: 1 in, 1 out]
                    n382 = Number To Fractional String(number=w772) -> (F-format string=w793:string)  [unwired: 3 in]
                    n383 = Fract/Exp String To Number(string=w769) -> (number=w770:dbl)  [unwired: 3 in, 1 out]
                    n384 = Increment(x=w778) -> (x+1=w798:i32)
                    n385 = call "LineScan量測值轉換.vi"("位數"=6, "input string"=w793, "PLC address"=20) -> ("error out"=w795:errorcluster)  [unwired: 7 in, 1 out]
                    n386 = Select(t=w798, s=w808, f=w798) -> (s? t:f=w809:i32)
                    n387 = Not(x=w808) -> (.not. x?=w771:bool)
                    n388 = case shown="True" w773 {
                      tunnel: w770 -> [_ w817]
                      tunnel: [w813 w816] -> w765
                      tunnel: w771 -> [w813 _]
                      frame False {
                      }
                      frame True {
                        n389 = call "ProjectSearchDataName.vi"("element"="$Voltage Up") -> ("variant"=w822:variant)  [unwired: 7 in, 3 out]
                        n390 = call "ProjectSearchDataName.vi"("element"="$Voltage Dn") -> ("variant"=w821:variant)  [unwired: 7 in, 3 out]
                        n391 = Variant To Data(type=0.0, Variant=w822) -> (data=w819:dbl)  [unwired: 1 in, 1 out]
                        n392 = Variant To Data(type=0.0, Variant=w821) -> (data=w818:dbl)  [unwired: 1 in, 1 out]
                        n393 = In Range and Coerce(upper limit=w819, x=w817, lower limit=w818) -> (In Range?=w816:bool)  [unwired: 1 out]
                      }
                    }
                    n394 = Greater Or Equal?(x=w809, y=w811) -> (x >= y?=w807:bool)
                    n395 = case shown="True" w807 {
                      tunnel: [errorcluster {"status"=FALSE, "code"=0, "source"=""} ("error constant") errorcluster {"status"=TRUE, "code"=18206, "source"=""} ("error constant")] -> w794
                      tunnel: w809 -> [w847 _]
                      tunnel: [w847 0] -> w777
                      tunnel: w806 -> [_ _]
                      frame False {
                      }
                      frame True {
                      }
                    }
                    n396 = Increment(x=w801) -> (x+1=w812:i32)
                    n397 = Merge Errors(w795, w794) -> (w766:errorcluster)
                    n398 = global read "Main Glb.vi" "Input Registers0-99"() -> (w781:u16[])
                    n399 = Select(t=w812, s=w765, f=w801) -> (s? t:f=w800:i32)
                    n400 = Select(t=w769, s=w765, f="NG" ("DataIn")) -> (s? t:f=w788:string)
                    n401 = case shown="No Error" w766 {
                      tunnel: [w825 w844] -> w780
                      tunnel: w765 -> [w824 _]
                      frame No Error {
                        n402 = case shown="True" w824 {
                          tunnel: [_ w830] -> w825
                          frame False {
                          }
                          frame True {
                            w831 = T5[] [enum."給PLC要量電壓訊號"] items=["S2站PC動作中_20", "電流量測完成產品OK_21", "電流量測完成產品NG_22", "S2站Format 執行_23", "S2 Format OK_24", "S2 Format NG_25", "S2站燒入執行_26", "S2站燒入OK_27", "S2站燒入NG_28", "S2站動作完成_29", "S3 PC動作中_30", "S3 Format 此站執行_31", "S3 Format OK_32", "S3 Format NG_33", "S3 燒入程式 此站執行_34", "S3 燒入程式 OK_35", "S3 燒入程式 NG_36", "S3 備用_37", "S3 備用_38", "S3 動作完成_39", "S4 PC動作中_40", "S4 量測完成 產品正常_41", "S4 量測完成 產品NG_42", "S4 Format 此站執行_43", "S4 Format OK_44", "S4 Format NG_45", "S4 燒入 此站不執行_46", "S4 燒入程式 OK_47", "S4 燒入程式 NG_48", "S4 藍芽Scan OK_49", "S4 藍芽Scan NG_50", "S4 動作完成_51", "給PLC要量電流訊號", "給PLC要量電壓訊號"]
                            w837 = T5[] [enum."S4 量測完成 產品正常_41"] items=["S2站PC動作中_20", "電流量測完成產品OK_21", "電流量測完成產品NG_22", "S2站Format 執行_23", "S2 Format OK_24", "S2 Format NG_25", "S2站燒入執行_26", "S2站燒入OK_27", "S2站燒入NG_28", "S2站動作完成_29", "S3 PC動作中_30", "S3 Format 此站執行_31", "S3 Format OK_32", "S3 Format NG_33", "S3 燒入程式 此站執行_34", "S3 燒入程式 OK_35", "S3 燒入程式 NG_36", "S3 備用_37", "S3 備用_38", "S3 動作完成_39", "S4 PC動作中_40", "S4 量測完成 產品正常_41", "S4 量測完成 產品NG_42", "S4 Format 此站執行_43", "S4 Format OK_44", "S4 Format NG_45", "S4 燒入 此站不執行_46", "S4 燒入程式 OK_47", "S4 燒入程式 NG_48", "S4 藍芽Scan OK_49", "S4 藍芽Scan NG_50", "S4 動作完成_51", "給PLC要量電流訊號", "給PLC要量電壓訊號"]
                            n403 = global read "Process Global.vi" "S2Tool Action"() -> (w829:bool[])
                            n404 = Replace Array Subset(array=w829, new element=TRUE ("new element/subarray"), index=5) -> (w826:bool[])
                            n405 = call "Set OutputPLC.vi"("Address In"=20, "Array 2"=w837, "Sat Coils"=bool[] [TRUE]) -> ("Error Out"=w836:errorcluster[])  [unwired: 7 in]
                            n406 = global write "Process Global.vi" "S2Tool Action"(w826) -> ()
                            n407 = Merge Errors(w836) -> (w835:errorcluster)
                            n408 = call "Set OutputPLC.vi"("Address In"=20, "Array 2"=w831, "Sat Coils"=bool[] [FALSE], "error in (no error)"=w835) -> ("Error Out"=w830:errorcluster[])  [unwired: 6 in]
                          }
                        }
                      }
                      frame Error {
                        w846 = T5[] [enum."S4 量測完成 產品NG_42"] items=["S2站PC動作中_20", "電流量測完成產品OK_21", "電流量測完成產品NG_22", "S2站Format 執行_23", "S2 Format OK_24", "S2 Format NG_25", "S2站燒入執行_26", "S2站燒入OK_27", "S2站燒入NG_28", "S2站動作完成_29", "S3 PC動作中_30", "S3 Format 此站執行_31", "S3 Format OK_32", "S3 Format NG_33", "S3 燒入程式 此站執行_34", "S3 燒入程式 OK_35", "S3 燒入程式 NG_36", "S3 備用_37", "S3 備用_38", "S3 動作完成_39", "S4 PC動作中_40", "S4 量測完成 產品正常_41", "S4 量測完成 產品NG_42", "S4 Format 此站執行_43", "S4 Format OK_44", "S4 Format NG_45", "S4 燒入 此站不執行_46", "S4 燒入程式 OK_47", "S4 燒入程式 NG_48", "S4 藍芽Scan OK_49", "S4 藍芽Scan NG_50", "S4 動作完成_51", "給PLC要量電流訊號", "給PLC要量電壓訊號"]
                        n409 = global read "Process Global.vi" "S2Tool Action"() -> (w843:bool[])
                        n410 = Replace Array Subset(array=w843, new element=FALSE ("new element/subarray"), index=5) -> (w840:bool[])
                        n411 = global write "Process Global.vi" "S2Tool Action"(w840) -> ()
                        n412 = call "Set OutputPLC.vi"("Address In"=20, "Array 2"=w846, "Sat Coils"=bool[] [TRUE]) -> ("Error Out"=w844:errorcluster[])  [unwired: 7 in]
                      }
                    }
                    n413 = call "Red PLC InReg.vi"("length"=10, "index"=20, "Input Registers Arr"=w781) -> ("Rad In Reg"=w782:string)  [unwired: 7 in, 1 out]
                    n414 = call "Cub Meaasure FGV.vi"("Action"=Table_Save."Write" ("Enum"), "Save Index"=MeasureDisplayTab."電池負載電壓", "DataIn"=w788, "SN"=w782) -> ()  [unwired: 8 in, 8 out]
                    n415 = Merge Errors(w780, w766) -> (w779:errorcluster)
                  }
                }
              }
            }
          }
          frame True {
            w851 = 0
          }
        }
        n416 = property class="DigNum (strict)"(reference=w51, "Value"=w52) -> ()  [unwired: 1 in, 2 out]
        n417 = disable-structure shown="Disabled" {
          disable-tunnel: w46 -> [w73 w76]
          disable-tunnel: [w72 w76] -> w45
          frame Disabled {
            n418 = call "ErrorCycleNoSet.vi"("error in"=w73, "CaseNo"=enum16{"S2", "S3", "S4", "S11"}."S2", "Error Set Item"="$AlarmCycleNo_S2") -> ("error out"=w72:errorcluster)  [unwired: 8 in]
          }
          frame Enabled {
          }
        }
        n419 = call "Exit.vi"() -> ("ExitOut"=w47:bool)  [unwired: 11 in]
        n420 = Compound Arithmetic op=OR(w46, w56, w47) -> (w67:bool)
        n421 = case shown="No Error" w46 {
          frame No Error {
            n422 = global write "Process Global.vi" "S2 OK"(TRUE ("S2 OK")) -> ()
          }
          frame Error {
            n423 = global write "Process Global.vi" "S2 NG"(TRUE ("S2 NG")) -> ()
          }
        }
        "present" <- w55
      }
    }
    frame Error {
    }
  }
  n424 = disable-structure shown="Disabled" {
    frame Disabled {
      n425 = case shown="True" {
        selector: _ -> [_ _]
        tunnel: [errorcluster {"status"=FALSE, "code"=0, "source"=""} ("error constant") w872] -> _
        tunnel: _ -> [_ w866]
        tunnel: [ProjectStepSelect."MToolWork" ("select step") w877] -> _
        tunnel: _ -> [_ w874]
        tunnel: _ -> [_ w869]
        tunnel: _ -> [_ w862]
        tunnel: [_ w861] -> _
        frame False {
          # "Format 先不驗證"
          n426 = call "Auto Inspection_Status.vi"("Action"=enum16{"Initial", "Write", "Read"}."Write", "DataIn"="Format Pass", "Station"=Auto_Inspection_Station_Name2."S2Measure", "Data"=Auto_Inspection_Data_Name."ItemSN(TimeCode)") -> ()  [unwired: 9 in, 3 out]
        }
        frame True {
          w875 = T14[] [enum."commamd1", enum."commamd2", enum."commamd3"] items=["Project Name", "commamd1", "commamd2", "commamd3", "wat time1", "return1", "return2", "return3", "wat time2", "over time", "retry"] ("Cmd Step")
          n427 = call "Project Cmd Combin.vi"("Cmd Step"=w875, "Content Input"=w874) -> ("concatenated string"=w876:string)  [unwired: 7 in, 2 out]
          n428 = call "Tool RS232 test.vi"("Cmd In"=w876, "VISA resource name"=refnum<visa-resource-name> "COM3", "action"=w866) -> ("error out"=w873:errorcluster, "receive string"=w870:string)  [unwired: 7 in]
          n429 = Match Pattern(string=w870, regular expression=w869) -> (offset past match=w868:i32)  [unwired: 1 in, 3 out]
          n430 = case shown="Error .." w873 {
            tunnel: [errorcluster {"status"=FALSE, "code"=0, "source"=""} ("error constant") errorcluster {"status"=TRUE, "code"=11500, "source"=""} ("error constant")] -> w872
            frame No Error {
            }
            frame Error {
            }
          }
          n431 = Greater Or Equal To 0?(x=w868) -> (x >= 0?=w863:bool)
          n432 = Unbundle By Name(w873) -> ("status"=w880:bool)
          n433 = Increment(x=w862) -> (x+1=w864:dbl)
          n434 = Not(x=w880) -> (.not. x?=w879:bool)
          n435 = Increment(x=w866) -> (x+1=w867:dbl)
          n436 = Select(t=w867, s=w863, f=w866) -> ()  [unwired: 1 out]
          n437 = Select(t=ProjectStepSelect."MToolWork" ("select step"), s=w879, f=ProjectStepSelect."Format" ("select step")) -> (s? t:f=w877:T13)
          n438 = Select(t=w862, s=w863, f=w864) -> (s? t:f=w861:dbl)
        }
      }
    }
    frame Enabled {
    }
  }
  n439 = disable-structure shown="Disabled" {
    frame Disabled {
      n440 = call "ModbusCmdIn.vi"("Enum"=ModbusCmd."Fetch Discrete Inputs") -> ()  [unwired: 10 in, 1 out]
    }
    frame Enabled {
    }
  }
  n441 = disable-structure shown="Disabled" {
    frame Disabled {
      # "收尋S2站條碼"
      n442 = call "ProjectSearchDataName.vi"("element"="$Voltage Dn") -> ("variant"=w891:variant)  [unwired: 7 in, 3 out]
      n443 = call "ProjectSearchDataName.vi"("element"="$ForceSetBinChk_") -> ("variant"=w889:variant)  [unwired: 7 in, 3 out]
      n444 = Variant To Data(type=0.0, Variant=w891) -> (data=→"data":dbl)  [unwired: 1 in, 1 out]
      n445 = Variant To Data(type=FALSE, Variant=w889) -> (data=→"data 2":bool)  [unwired: 1 in, 1 out]
      n446 = Select(t="OK" ("DataIn"), f="NG" ("DataIn")) -> (s? t:f=w892:string)  [unwired: 1 in]
      n447 = global read "Main Glb.vi" "Input Registers0-99"() -> (w899:u16[])
      n448 = call "Red PLC InReg.vi"("length"=10, "index"=20, "Input Registers Arr"=w899) -> ("Rad In Reg"=w898:string)  [unwired: 7 in, 1 out]
      n449 = call "Cub Meaasure FGV.vi"("Action"=Table_Save."Write" ("Enum"), "Save Index"=MeasureDisplayTab."Programe(Tool Programe)", "DataIn"=w892, "SN"=w898) -> ()  [unwired: 5 in, 7 out]
    }
    frame Enabled {
    }
  }
  n450 = call "ErrorCycleNoSet.vi"("error in"=w2, "CaseNo"=enum16{"S2", "S3", "S4", "S11"}."S2", "Error Set Item"="$AlarmCycleNo_S2") -> ("error out"=w1:errorcluster)  [unwired: 8 in]
  "error out" <- w1
  n451 = disable-structure shown="Disabled" {
    disable-tunnel: w1 -> [w901 _]
    frame Disabled {
      n452 = case shown="No Error" w901 {
        frame No Error {
          n453 = global write "Process Global.vi" "S2 OK"(TRUE ("S2 OK")) -> ()
        }
        frame Error {
          n454 = global write "Process Global.vi" "S2 NG"(TRUE ("S2 NG")) -> ()
        }
      }
    }
    frame Enabled {
    }
  }
  n455 = Select(t=Station_Action."Dectect Action" ("Station Out"), s=w1, f=Station_Action."ImformOut" ("Station Out")) -> (s? t:f=→"Station Out":T1)
  "LineScan out" <- "LineScan in"
